vi "MegaAwesome_9_21_12c_JW.vi"() -> ()   [LabVIEW 2011]
uses:
  MegaAwesome_States.ctl
  <vilib>/Utility/inputDevices.llb/keyboardAcquire.vi
  <vilib>/Utility/file.llb/Read From Spreadsheet File (string).vi
  <vilib>/Utility/file.llb/Write To Spreadsheet File (string).vi
panel:
  out "Image Center X":i32
  in  "Disable Flag":bool
  out "Index":string
  out "ROI Descriptor out":T1 {"Contours"."Type" items=["No Selection", "Point", "Line", "Rectangle", "Oval", "Polygon", "Freehand Region", "Annulus", "Unused2", "Unused3", "Broken Line", "Freehand Line", "Rotated Rectangle"]}
  out "ROI Descriptor":T1 {"Contours"."Type" items=["No Selection", "Point", "Line", "Rectangle", "Oval", "Polygon", "Freehand Region", "Annulus", "Unused2", "Unused3", "Broken Line", "Freehand Line", "Rotated Rectangle"]}
  in  "Slider Min":dbl=5.0
  in  "Slider Max":dbl=5.0
  out "Opj X Axis":string
  out "X Axis Display Type":string
  in  "Index-Sat":dbl=5.0
  in  "Index-Lin":dbl=5.0
  in  "IndexLog-Lin":dbl=5.0
  in  "IndexLog-Sat":dbl=5.0 caption="Num Pts"
  out "Lin Id-Log Used":dbl[](array[numeric])
  out "Lin-Vg Array-Log Used":dbl[](array[numeric])
  in  "New: Comments":string
  out "Save Array":string[][](array[string])
  out "Folder Index":i32 caption="Length"
  out "Sat Id-Used":dbl[](array[numeric])
  out "Sat Vg Array-Used":dbl[](array[numeric])
  out "Vg Array-Log-Used":dbl[](array[numeric])
  out "Sat Id-Log-Used":dbl[](array[numeric])
  out "Lin Id-Used":dbl[](array[numeric])
  out "Lin-Vg Array-Used":dbl[](array[numeric])
  out "Lin Vd":dbl
  out "Recorded Prop":T2
  out "Current State":T3
  in  "Main Tab Control":T4(tab)
  in  "1) Transport":bool caption="2) Transport"
  in  "Image Analysis":bool caption="1) Image Analysis"
  in  "Transport\nFolder":path caption="Transport Folder"
  out "Transport\nFile":path=path "D:/UserData/Desktop/Jeremy/WFU/Research/Programs/VI mods/Image Not Found.png" caption="Transport File"
  in  "Image Folder":path
  out "Image File":path=path "D:/UserData/Desktop/Jeremy/WFU/Research/Programs/VI mods/Image Not Found.png"
  in  "Transfer File":path
  out "Transfer Folder":path
  out "Fabrication Prop":T5
  out "Distances":dbl[](array[numeric])
  in  "Zoom":i16(slide)=-3 scale=-5.0..5.0
  in  "Magnification":u16(ring) items=["5x", "10x", "20x", "50x", "80x"]
  in  "Undo Button":bool
  in  "Remove Button":bool
  in  "Transfer Plots":T6(tab)=enum."Saturation"
  in  "Lin-Trans Slider":dbl(slide) step=1.0 scale=-40.0..40.0 scale format="%#_1p"
  out "Sqrt-Lin":cluster{dbl[], dbl[]}[](graph)
  in  "Sat-Trans Slider":dbl(slide) step=1.0 scale=-40.0..40.0 scale format="%#_1p"
  out "Sqrt-Sat":cluster{dbl[], dbl[]}[](graph)
  out "Raw- Lin":cluster{dbl[], dbl[]}[](graph)
  out "Raw- Sat":cluster{dbl[], dbl[]}[](graph)
  in  "Log Plots":enum32{"Linear", "Saturation", "Transport"}(tab)=enum."Saturation"
  in  "Lin-Log Slider":dbl(slide) step=1.0 scale=-40.0..40.0 scale format="%#_1p"
  out "Log-Lin":cluster{dbl[], dbl[]}[](graph)
  in  "Sat-Log Slider":dbl(slide) step=1.0 scale=-40.0..40.0 scale format="%#_1p"
  out "Sat-Log":cluster{dbl[], dbl[]}[](graph)
  out "Transport":cluster{dbl[], dbl[]}[](graph)
  out "Transport Name:":string
  in  "Manual Controls":T7
  in  "File Controls":T8
  out "Date Recorded":string="Date Recorded" caption="Measured"
  out "Data Name:":string
  out "Image Name":string
  out "Date Created":string caption="Fabricated"
  in  "Comments:":string
  out "Rec: Length":dbl caption="Length" format="%#_3g"
  out "Rec: Width":dbl caption="Width" format="%#_4g"
  out "Rec: Dielectric (d)":dbl caption="Dielectric (d)" format="%#_3g"
  in  "New: Dielectric":dbl
  in  "New: Length":dbl
  in  "New: Width":dbl
  out "Rec: Temp":dbl caption="Sample Temp" format="%.1f"
  in  "New: Temp":dbl format="%.1f"
  out "Image Out":T9(plugin-control)
  in  "Num Pts":dbl=5.0
  in  "Num Pts Log":dbl=5.0 caption="Num Pts"
  out "Recorded Values Cluster":T10
  out "Calculated Values Cluster":T10 caption="Recorded Values Cluster"
  out "Re-Calculated Values Cluster":T10 caption="Recorded Values Cluster"
  in  "Independant Variable:":string(combo)="Length (um):"
  out "Image Preview":T9(plugin-control)
  out "Total Width":dbl
  in  "Index Array":u16(ring) caption="Index" items=["X 1B", "X 1C", "X 1D", "X 1E", "X 1F", "X 1H", "X 1J", "X 2A", "X 2B", "X 2C", "X 2D", "X 2E", "X 2F", "X 2G", "X 2H", "X 2J", "X 3A", "X 3B", "X 3C", "X 3D", "X 3E", "X 3F", "X 3G", "X 3H", "X 3J", "X 4A", "X 4B", "X 4C", "X 4D", "X 4E", "X 4F", "X 4G", "X 4H", "X 4J", "X 5A", "X 5B", "X 5C", "X 5D", "X 5E", "X 5F", "X 5G", "X 5H", "X 5J", "X 6A", "X 6B", "X 6C", "X 6D", "X 6E", "X 6F", "X 6G", "X 6H", "X 6J", "X 7A", "X 7B", "X 7C", "X 7D", "X 7E", "X 7F", "X 7G", "X 7J", "X 8A", "X 8B", "X 8C", "X 8D", "X 8E", "X 8F", "X 8G", "X 8H", "X 8J", "X 9C", "X 9D", "X F_"]
  in  "Room Temp":dbl=294.0 caption="Room Temp (K)"
  in  "No Image\n File":path=path "\\\\acad1\\physics/Jurchescu-group/JW-PD/Mega Awesome/Image Not Found.png" caption="No Image File"
  in  "Origin Project File":path=path "\\\\acad1\\physics/Jurchescu-group/JW-PD/Group Library/Origin Project Files/DeviceData_8_10_12a_JW.opj"
  in  "No Transport\n File":path=path "\\\\acad1\\physics/Jurchescu-group/JW-PD/Mega Awesome/No Transport File.txt" caption="No Transport File"
  in  "Transport Style Controls":T11={"Transport Line Size"=1, "Transport Line Color"=16772608} {"Transport Line Size" items=["Extra Small", "Small", "Medium", "Large", "Extra Large"]}
  # "Transfer Location"
  # "What else would you like to view during your analysis?"
  # "Image Location"
  # "Transport Location"
  # "Recorded"
  # "Calculated"
  # "Re-Calculated"
  # "Manual"
  # "Used points display at y=0\nValues are wrong w/ slider"
  # "Slider\nDoesn't\nWork"
  # "Slider\nDoesn't\nWork"
  # "No new points displayed"
  # "Default File Choices"
  # "Default Analysis Values"
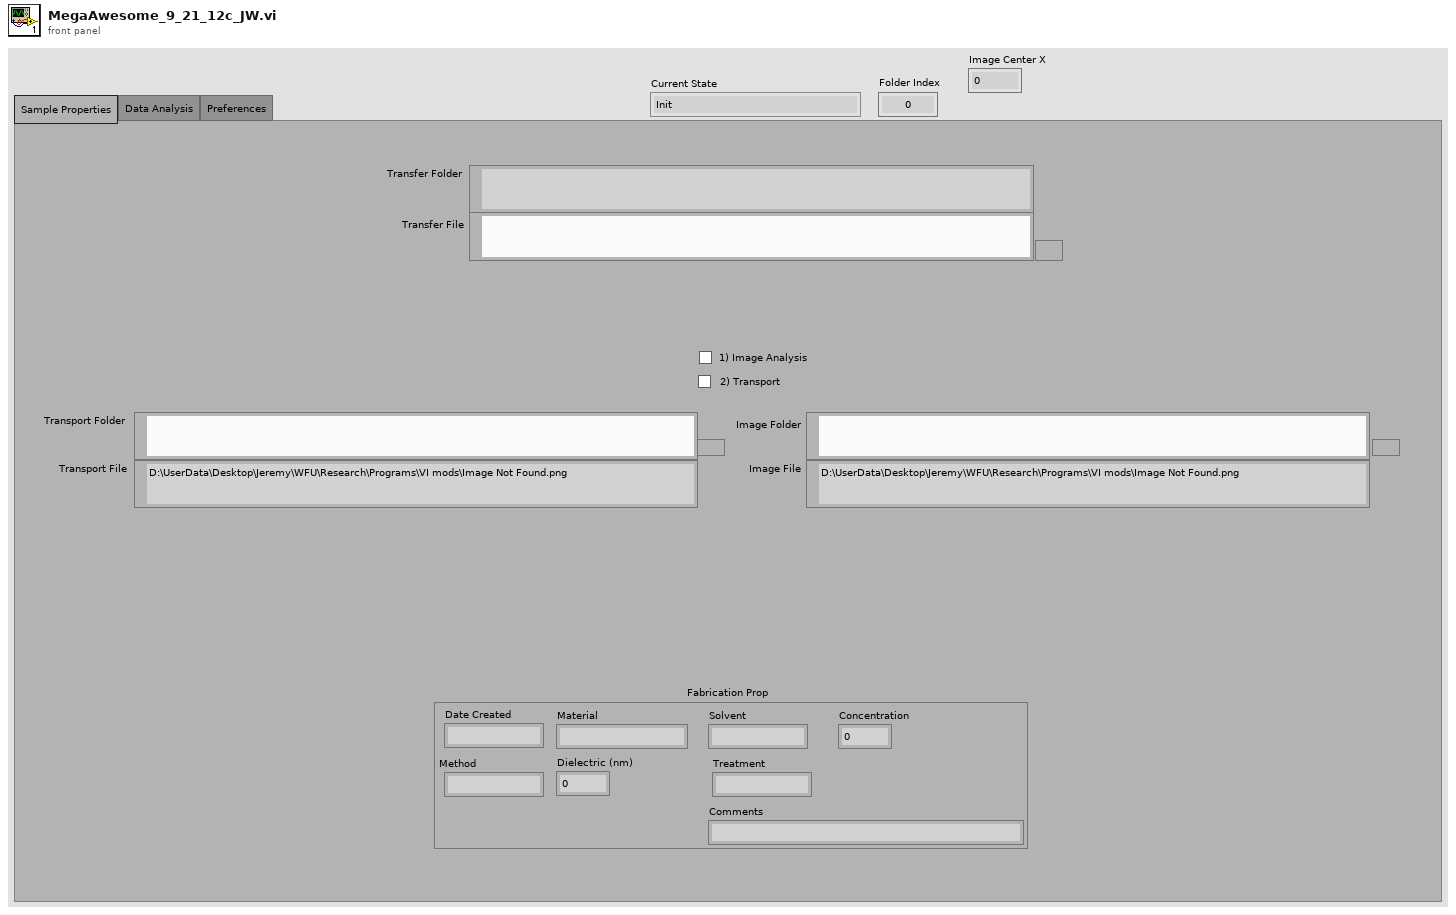
[diagram p1: front panel]
types:
  T1 = typedef "ROI Descriptor" = cluster{"Global Rectangle":i32[], "Contours":cluster{"ID":enum32{"External", "Internal"}, "Type":u32, "Coordinates":i32[]}[]}
  T2 = cluster{"Date Recorded":string, "Index":string, "Length":dbl, "Width":dbl, "Sample Temp":dbl}
  T3 = typedef "MegaAwesome_States.ctl" = enum16{"Init", "File Missing", "No Event", "Read Data", "Calculated Values", "Re-Calculated Values", "Next File", "Previous File", "Discard File", "Save", "Save Lines", "Export", "Exit"}
  T4 = enum32{"Sample Properties", "Data Analysis", "Preferences"}
  T5 = cluster{"Date Created":string, "Material":string, "Solvent":string, "Concentration":dbl, "Method":string, "Dielectric (nm)":dbl, "Treatment":string, "Comments":string}
  T6 = enum32{"Linear", "Saturation", "Raw-Linear", "Raw-Saturation"}
  T7 = cluster{"Manual-Temp":bool, "Manual-Width":bool, "Manuel-Length":bool, "Manuel-Dielectric":bool, "Manual Comments":bool}
  T8 = cluster{"Previous File":bool, "Discard ":bool, "Save Lines":bool, "Close":bool, "Next File ":bool, "Save":bool, "Save Next":bool, "Export":bool}
  T9 = typedef "IMAQ Image.ctl" = refnum<image>
  T10 = cluster{"Mobility-Sat":dbl, "Moblitity-Lin":dbl, "On/Off":dbl, "Off Current":dbl, "Vt-Sat":dbl, "STS":dbl, "Trap Density-VT":dbl, "Trap Density-STS":dbl}
  T11 = cluster{"Transport Line Size":u16, "Transport Line Color":u32}
  T12 = typedef "LVBoundsTypeDef.ctl" = cluster{"Width":u32, "Height":u32}
  T13 = cluster{"Global Rectangle":i32[], "Contours":cluster{"Contour Type":u32, "ROI Type":u32, "Points":i32[]}[]}
  T14 = cluster{"Contour Type":u32, "ROI Type":u32, "Points":i32[]}[]
  T15 = cluster{i32[], cluster{"Contour Type":u32, "ROI Type":u32, "Points":i32[]}[]}
  T16 = enum16{"0", "1", "2", "3", "4", "5", "6", "7", "8", "9", "A", "B", "C", "D", "E", "F", "G", "H", "I", "J", "K", "L", "M", "N", "O", "P", "Q", "R", "S", "T", "U", "V", "W", "X", "Y", "Z", "F1", "F2", "F3", "F4", "F5", "F6", "F7", "F8", "F9", "F10", "F11", "F12", "F13", "F14", "F15", "ADD", "BACK", "BACKSLASH", "CAPITAL", "COMMA", "DECIMAL", "DELETE", "DIVIDE", "DOWN", "END", "EQUALS", "ESCAPE", "GRAVE (`)", "HOME", "INSERT", "LBRACKET", "LCONTROL", "LEFT", "L ALT", "LSHIFT", "LWIN", "MINUS", "MULTIPLY", "NEXT", "NUMLOCK", "NUMPAD_0", "NUMPAD_1", "NUMPAD_2", "NUMPAD_3", "NUMPAD_4", "NUMPAD_5", "NUMPAD_6", "NUMPAD_7", "NUMPAD_8", "NUMPAD_9", "PAUSE", "PERIOD", "PRIOR (PG UP)", "RBRACKET", "RCONTROL", "RETURN", "RIGHT", "R ALT", "RSHIFT", "RWIN", "SCROLL", "SEMICOLON", "SLASH", "SPACE", "SUBTRACT", "TAB", "UP", "ENTER (num pad)", "' (quote)"}[]
  T17 = enum16{"0", "1", "2", "3", "4", "5", "6", "7", "8", "9", "A", "B", "C", "D", "E", "F", "G", "H", "I", "J", "K", "L", "M", "N", "O", "P", "Q", "R", "S", "T", "U", "V", "W", "X", "Y", "Z", "F1", "F2", "F3", "F4", "F5", "F6", "F7", "F8", "F9", "F10", "F11", "F12", "F13", "F14", "F15", "ADD", "BACK", "BACKSLASH", "CAPITAL", "COMMA", "DECIMAL", "DELETE", "DIVIDE", "DOWN", "END", "EQUALS", "ESCAPE", "GRAVE (`)", "HOME", "INSERT", "LBRACKET", "LCONTROL", "LEFT", "L ALT", "LSHIFT", "LWIN", "MINUS", "MULTIPLY", "NEXT", "NUMLOCK", "NUMPAD_0", "NUMPAD_1", "NUMPAD_2", "NUMPAD_3", "NUMPAD_4", "NUMPAD_5", "NUMPAD_6", "NUMPAD_7", "NUMPAD_8", "NUMPAD_9", "PAUSE", "PERIOD", "PRIOR (PG UP)", "RBRACKET", "RCONTROL", "RETURN", "RIGHT", "R ALT", "RSHIFT", "RWIN", "SCROLL", "SEMICOLON", "SLASH", "SPACE", "SUBTRACT", "TAB", "UP", "ENTER (num pad)", "' (quote)"}
  T18 = cluster{string, sgl, bool, bool, bool, bool, bool, bool, i32}
  T19 = cluster{i32, cluster{string, sgl, bool, bool, bool, bool, bool, bool, i32}, i32, i32}
  T20 = cluster{"Contour Type":u32, "ROI Type":u32, "Points":i32[]}
  T21 = cluster{"Points[0]":i32, "Points[1]":i32, "Points[2]":i32, "Points[3]":i32, "Points[4]":i32, "Points[5]":i32, "Points[6]":i32, "Points[7]":i32, "Points[8]":i32}
  T22 = cluster{"[0]":cluster{dbl[], dbl[]}, "[1]":cluster{dbl[], dbl[]}, "[2]":cluster{dbl[], dbl[]}, "[3]":cluster{dbl[], dbl[]}, "[4]":cluster{dbl[], dbl[]}, "[5]":cluster{dbl[], dbl[]}, "[6]":cluster{dbl[], dbl[]}, "[7]":cluster{dbl[], dbl[]}, "[8]":cluster{dbl[], dbl[]}}
  T23 = cluster{"Sat Vg Used":dbl[], "Sat Sqrt(Id) Used ":dbl[], "Lin Vg Used":dbl[], "Lin Sqrt(Id) Used":dbl[], "Index-Lin":dbl, "Index-Sat":dbl}
  T24 = cluster{"Raw Sat":cluster{dbl[], dbl[]}[], "Sqrt Sat":cluster{dbl[], dbl[]}[], "Log Sat":cluster{dbl[], dbl[]}[], "Raw Lin":cluster{dbl[], dbl[]}[], "Sqrt Lin":cluster{dbl[], dbl[]}[], "Log Lin":cluster{dbl[], dbl[]}[]}
  T25 = cluster{"Mobility-Sat":dbl, "Vt-Sat":dbl, "Mobility-Lin":dbl, "Vt-Lin":dbl, "Off I-Sat":dbl, "On/Off I-Sat":dbl}
  T26 = cluster{"Sat Vg Used":dbl[], "Sat Log(Id) Used":dbl[], "Lin Vg Used":dbl[], "Lin Log(Id) Used":dbl[], "STS Index-Sat":dbl, "STS Index-Lin":dbl}
  T27 = cluster{"Independant  Variable Indicator":string, "Parameter String Indicator":string}
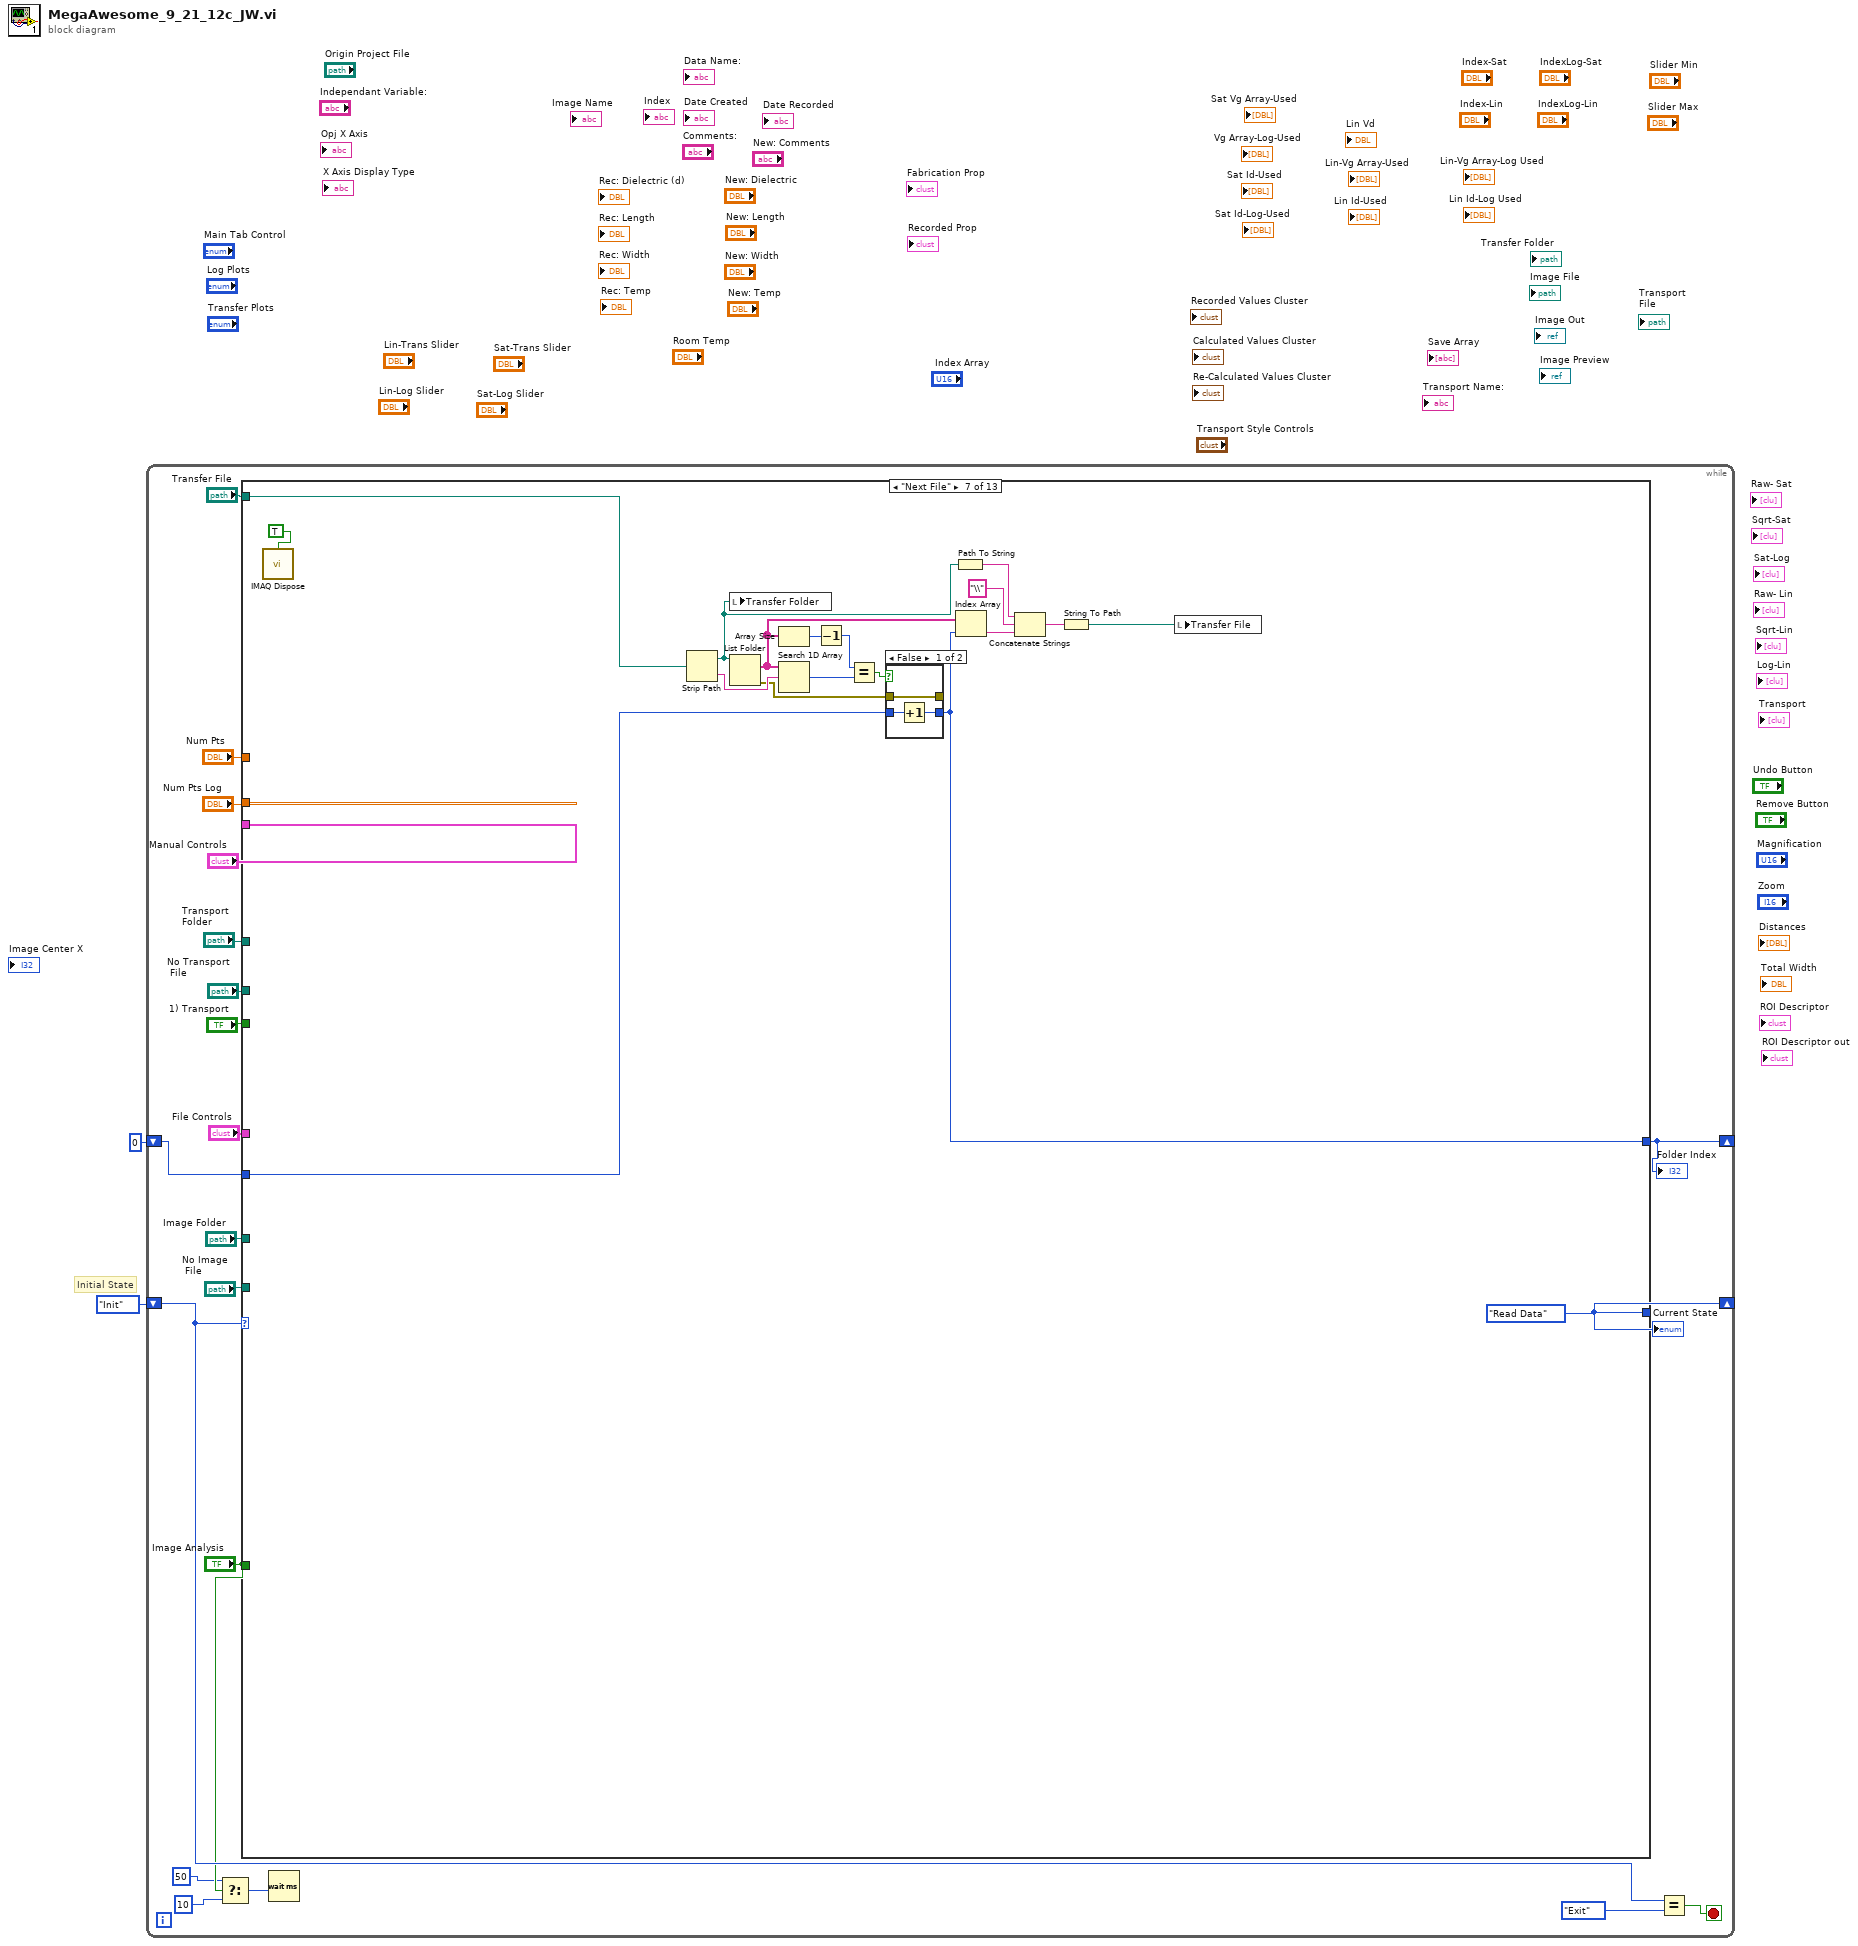
[diagram p0: block diagram]
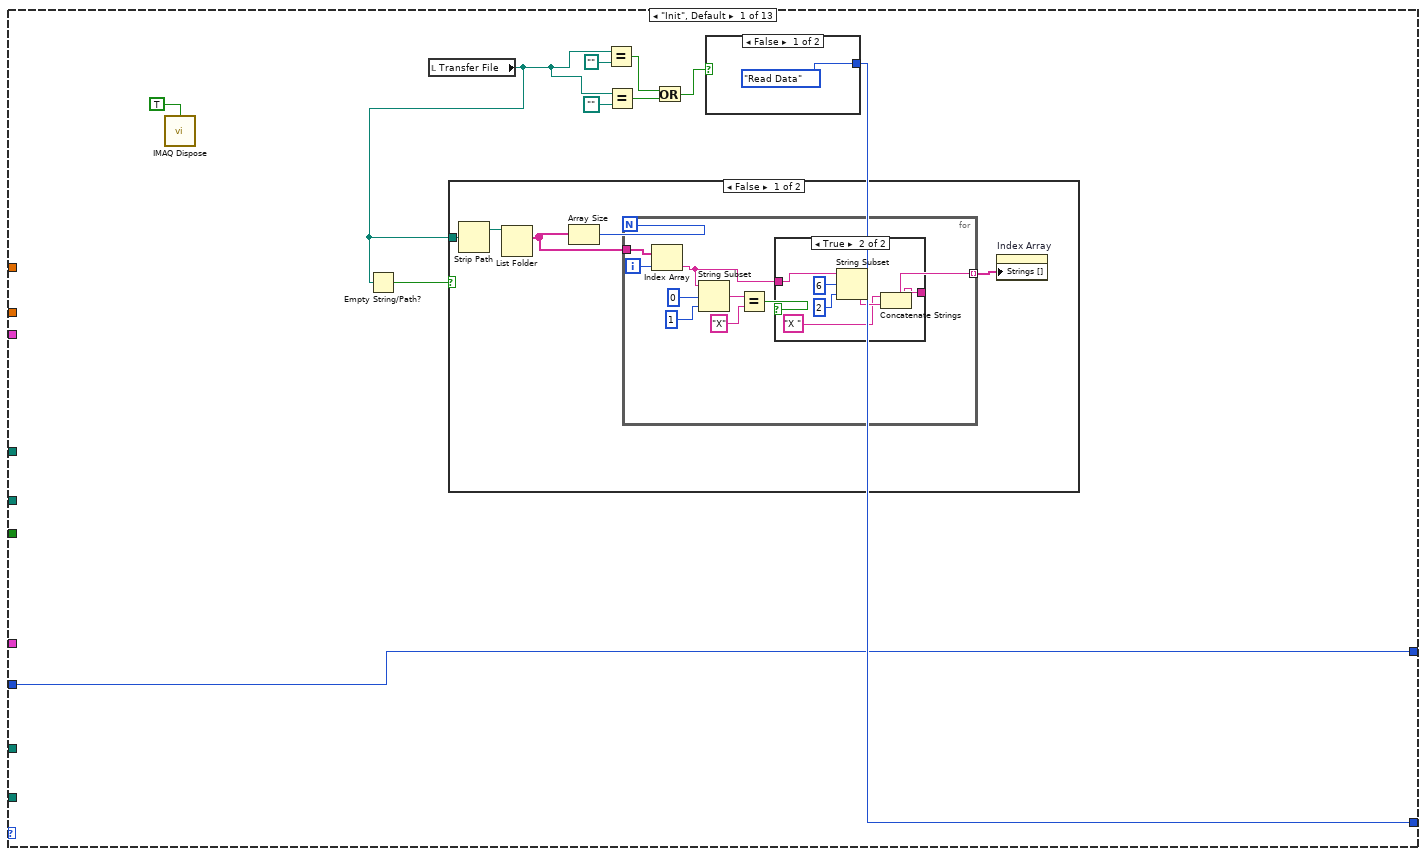
[diagram p2: hidden frame]
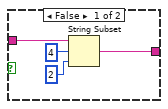
[diagram p3: hidden frame]
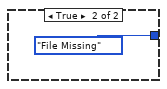
[diagram p5: hidden frame]
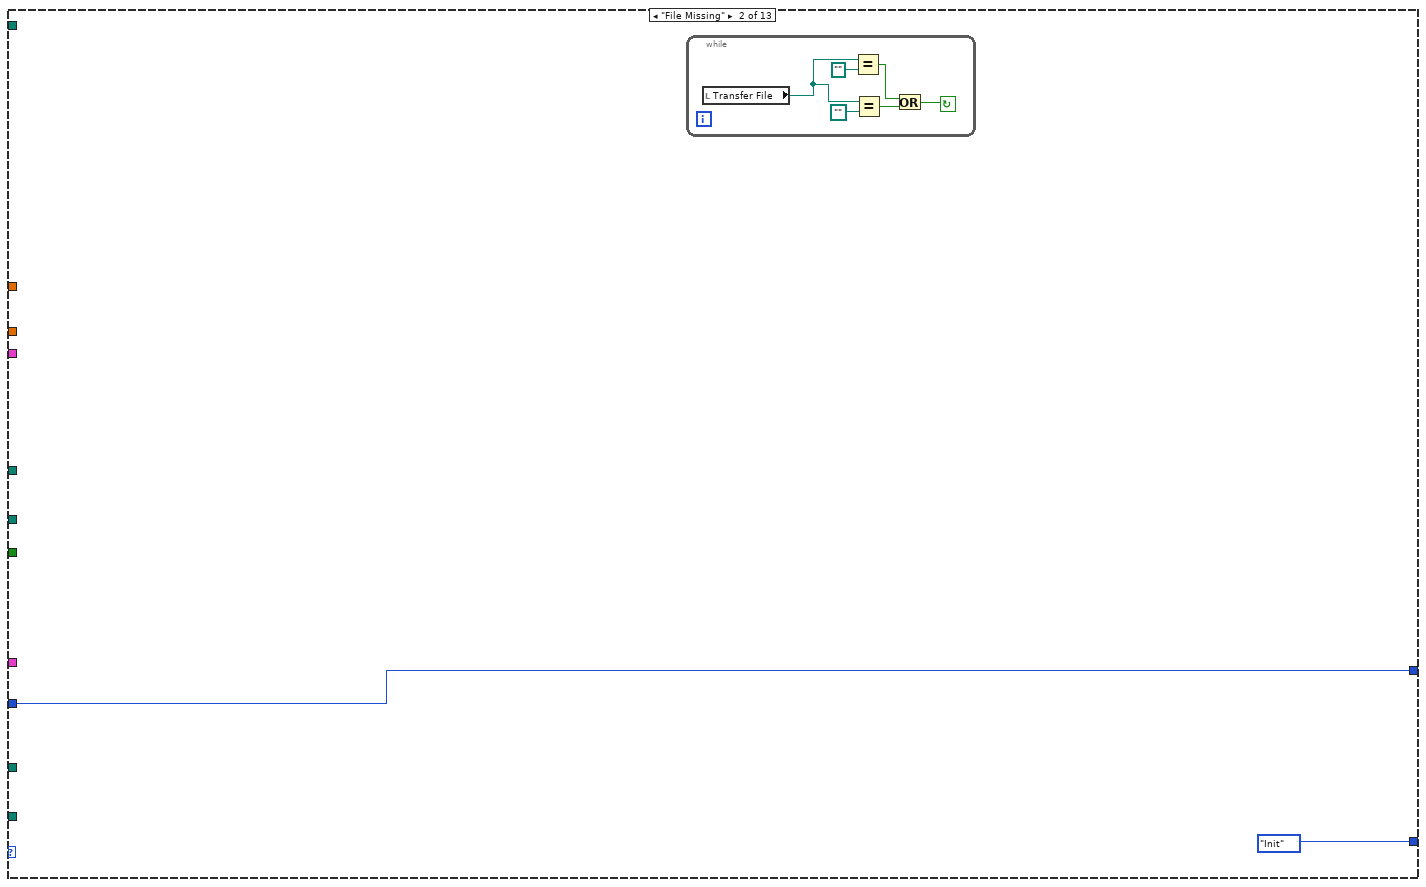
[diagram p6: hidden frame]
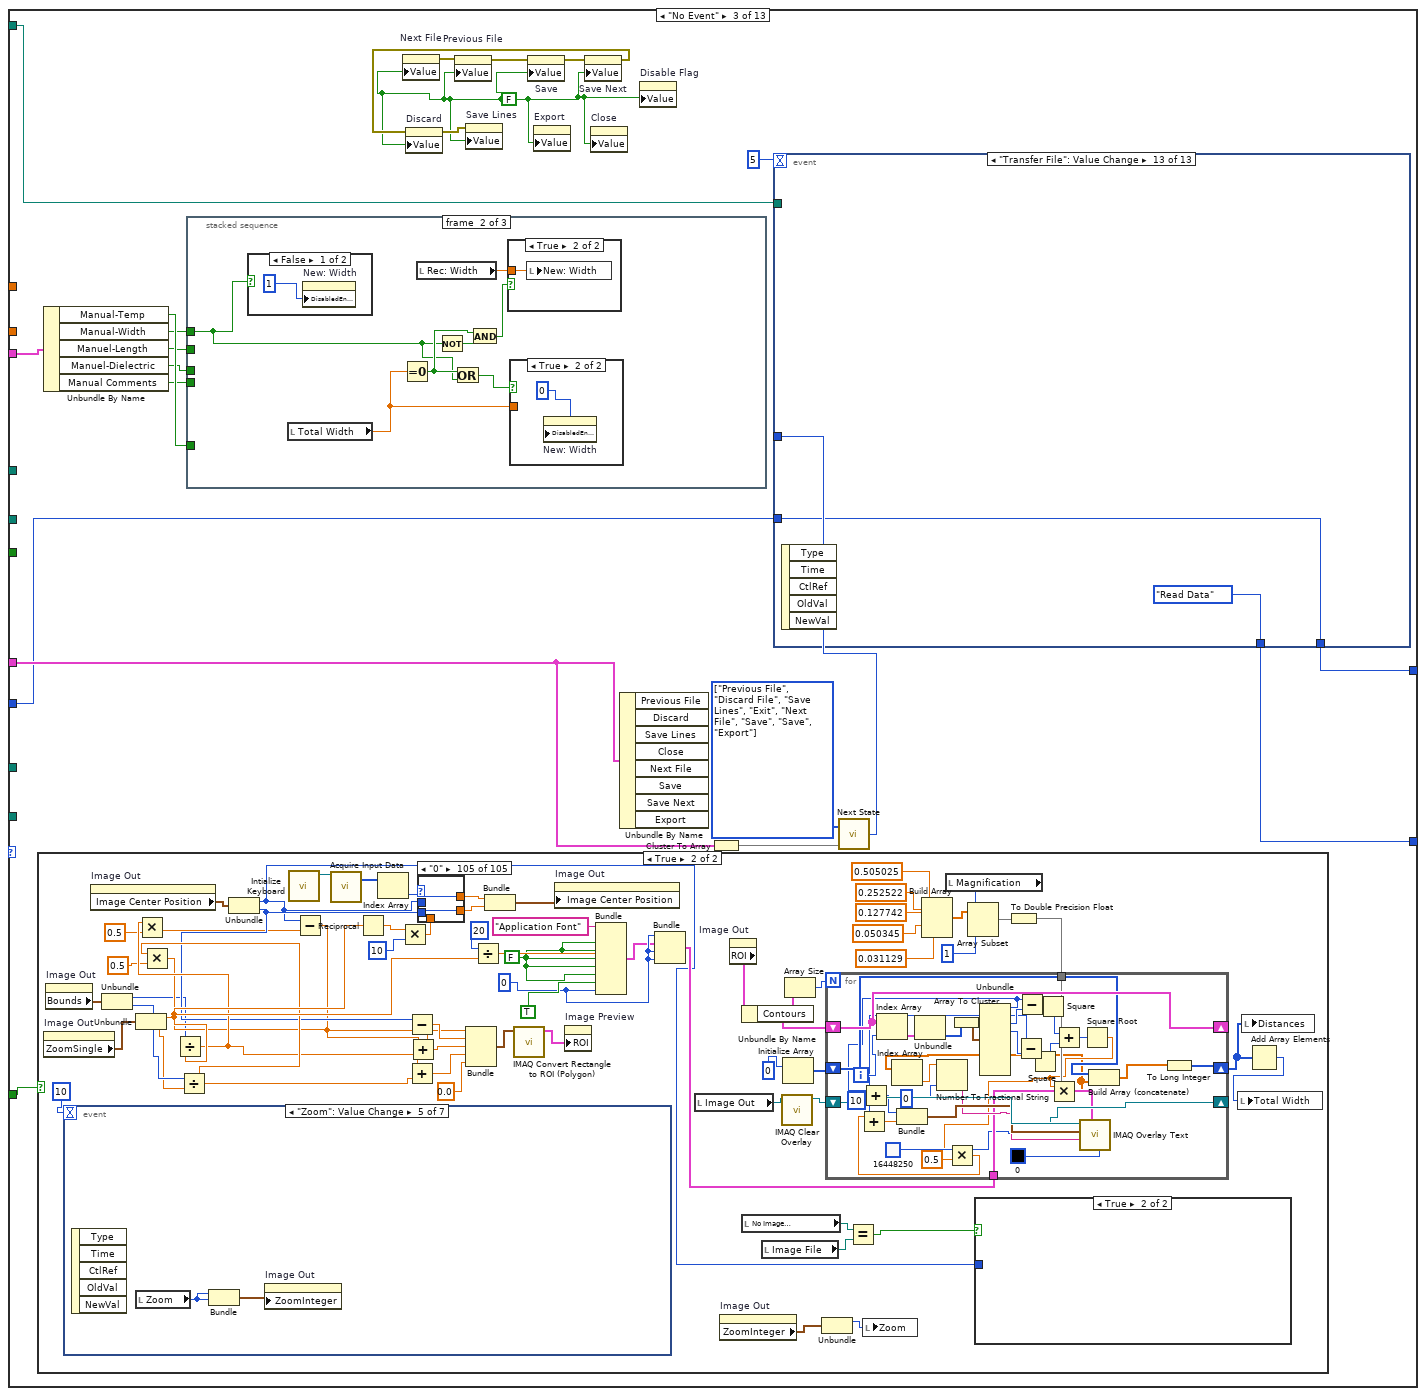
[diagram p7: hidden frame]
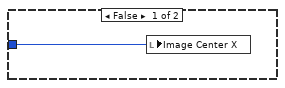
[diagram p9: hidden frame]
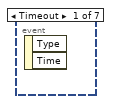
[diagram p10: hidden frame]
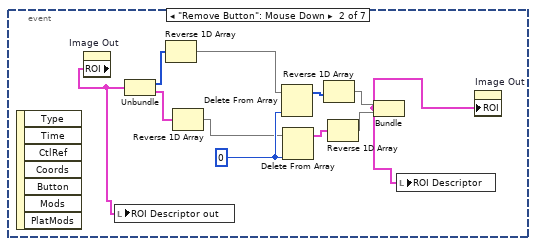
[diagram p11: hidden frame]
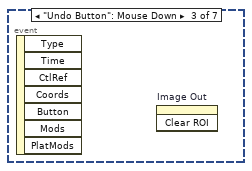
[diagram p12: hidden frame]
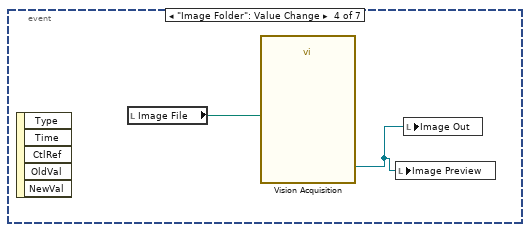
[diagram p13: hidden frame]
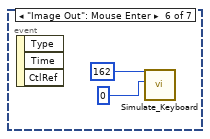
[diagram p14: hidden frame]
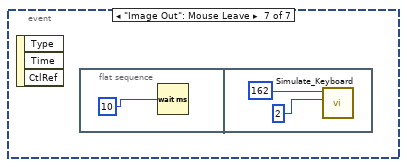
[diagram p15: hidden frame]
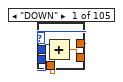
[diagram p16: hidden frame]
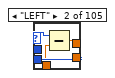
[diagram p17: hidden frame]
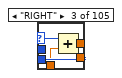
[diagram p18: hidden frame]
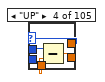
[diagram p19: hidden frame]
diagram:
  # "Initial State"
  n1 = while {
    shift-right: [w19] -> _
    shift-left: MegaAwesome_States."Init" -> [w21]
    shift-right: [w12] -> _
    shift-left: 0 -> [w13]
    stop <- w22 stop-if-true
    n2 = Select(t=50, s="Image Analysis", f=10) -> (s? t:f=w6:i32)
    n3 = case shown="\"Next File\"" w21 {
      tunnel: [w27 MegaAwesome_States."Init" w79 MegaAwesome_States."Calculated Values" MegaAwesome_States."Re-Calculated Values" MegaAwesome_States."No Event" MegaAwesome_States."Read Data" MegaAwesome_States."Read Data" MegaAwesome_States."Init" w813 MegaAwesome_States."No Event" MegaAwesome_States."No Event" MegaAwesome_States."Exit"] -> w19
      tunnel: "Transfer File" -> [_ _ w68 w578 w628 _ w750 w763 w784 w818 _ _ _]
      tunnel: "Num Pts" -> [_ _ _ _ w652 _ _ _ _ _ _ _ _]
      tunnel: "Num Pts Log" -> [_ _ _ _ w651 _ _ _ _ _ _ _ _]
      tunnel: "Image Folder" -> [_ _ _ _ w648 _ _ _ _ _ _ w1337 _]
      tunnel: "No Image\n File" -> [_ _ _ _ w647 _ _ _ _ _ _ _ _]
      tunnel: [w26 w59 w69 w583 w646 w709 w735 w761 w779 w819 w1334 w1347 w1351] -> w12
      tunnel: w13 -> [w26 w59 w70 w581 w646 w709 w736 w762 _ w819 w1334 w1347 w1351]
      tunnel: "Manual Controls" -> [_ _ w81 _ _ _ _ _ _ w817 _ _ _]
      tunnel: "File Controls" -> [_ _ w77 _ _ _ _ _ _ w812 _ _ _]
      tunnel: "1) Transport" -> [_ _ _ _ w618 _ _ _ _ _ _ _ _]
      tunnel: "Image Analysis" -> [_ _ w71 _ w617 _ _ _ _ _ _ _ _]
      tunnel: "Transport\nFolder" -> [_ _ _ _ w616 _ _ _ _ _ _ _ _]
      tunnel: "No Transport\n File" -> [_ _ _ _ w615 _ _ _ _ _ _ _ _]
      frame "Init", Default {
        n4 = call "IMAQ Dispose"("All Images? (No)"=TRUE) -> ()  [unwired: 5 in, 1 out]
        n5 = local read "Transfer File"() -> (w24:path)
        n6 = Empty String/Path?(string/path=w24) -> (empty?=w25:bool)
        n7 = case shown="False" w25 {
          tunnel: w24 -> [w34 _]
          frame False {
            n8 = Strip Path(path=w34) -> (stripped path=w36:path)  [unwired: 1 out]
            n9 = List Folder(path=w36) -> (filenames=w35:string[])  [unwired: 3 in, 3 out]
            n10 = Array Size(array=w35) -> (size(s)=w37:i32)
            n11 = for {
              N: w37 -> [_]
              tunnel: w35 -> [w46]
              tunnel: [w44] -> w33 mode=indexing
              i -> [w45]
              n12 = Index Array(array=w46, index=w45) -> (element=w43:string)
              n13 = String Subset(string=w43, offset (0)=0, length (rest)=1) -> (substring=w40:string)
              n14 = Equal?(x=w40, y="X") -> (x = y?=w39:bool)
              n15 = case shown="True" w39 {
                tunnel: w43 -> [w50 w54]
                tunnel: [w47 w53] -> w44
                frame False {
                  n16 = String Subset(string=w50, offset (0)=4, length (rest)=2) -> (substring=w47:string)
                }
                frame True {
                  n17 = String Subset(string=w54, offset (0)=6, length (rest)=2) -> (substring=w52:string)
                  n18 = Concatenate Strings("X ", w52) -> (w53:string)
                }
              }
            }
            n19 = property on="Index Array" class="Ring (strict)"("Strings []"=w33) -> ()  [unwired: 2 in, 2 out]
          }
          frame True {
          }
        }
        n20 = Equal?(x=w24, y=path "") -> (x = y?=w30:bool)
        n21 = Equal?(x=w24, y=path "") -> (x = y?=w29:bool)
        n22 = Or(x=w30, y=w29) -> (x .or. y?=w32:bool)
        n23 = case shown="False" w32 {
          tunnel: [MegaAwesome_States."Read Data" MegaAwesome_States."File Missing"] -> w27
          frame False {
          }
          frame True {
          }
        }
      }
      frame "File Missing" {
        n24 = while {
          stop <- w61 continue-if-true
          n25 = local read "Transfer File"() -> (w62:path)
          n26 = Equal?(x=w62, y=path "") -> (x = y?=w64:bool)
          n27 = Equal?(x=w62, y=path "") -> (x = y?=w65:bool)
          n28 = Or(x=w64, y=w65) -> (x .or. y?=w61:bool)
        }
      }
      frame "No Event" {
        w67 = FALSE
        w88 = T3[] [enum."Previous File", enum."Discard File", enum."Save Lines", enum."Exit", enum."Next File", enum."Save", enum."Save", enum."Export"] items=["Init", "File Missing", "No Event", "Read Data", "Calculated Values", "Re-Calculated Values", "Next File", "Previous File", "Discard File", "Save", "Save Lines", "Export", "Exit"]
        n29 = case shown="True" w71 {
          frame False {
          }
          frame True {
            w144 = FALSE
            w146 = 0
            n30 = property on="Image Out" class="ImageControl"() -> ("ZoomSingle"=w130:cluster{"X":sgl, "Y":sgl})  [unwired: 2 in, 2 out]
            n31 = property on="Image Out" class="ImageControl"() -> ("Bounds"=w129:T12)  [unwired: 2 in, 2 out]
            n32 = event shown="[4] \"Zoom\": Value Change" {
              selector: _ -> [_ _ _ _ _ _ _]
              dyn-events: _ -> [_ _ _ _ _ _ _]
              timeout: 10 -> [_ _ _ _ _ _ _]
              event Timeout {
                n33 = event-data() -> ()  [unwired: 1 in, 2 out]
              }
              event "Remove Button": Mouse Down {
                w164 = 0
                n34 = event-data() -> ()  [unwired: 1 in, 7 out]
                n35 = property on="Image Out" class="ImageControl"() -> ("ROI"=w154:T13)  [unwired: 2 in, 2 out]
                n36 = local write "ROI Descriptor out"(w154) -> ()
                n37 = Unbundle(w154) -> ("Global Rectangle"=w163:i32[], "Contours"=w161:T14)
                n38 = Reverse 1D Array(array=w163) -> (reversed array=w162:i32[])
                n39 = Reverse 1D Array(array=w161) -> (reversed array=w160:T14)
                n40 = Delete From Array(array=w162, index=w164) -> (array with subset deleted=w159:i32[])  [unwired: 1 in, 1 out]
                n41 = Delete From Array(array=w160, index=w164) -> (array with subset deleted=w158:T14)  [unwired: 1 in, 1 out]
                n42 = Reverse 1D Array(array=w159) -> (reversed array=w157:i32[])
                n43 = Reverse 1D Array(array=w158) -> (reversed array=w156:T14)
                n44 = Bundle(w157, w156) -> (w155:T15)  [unwired: 1 in]
                n45 = local write "ROI Descriptor"(w155) -> ()
                n46 = property on="Image Out" class="ImageControl"("ROI"=w155) -> ()  [unwired: 2 in, 2 out]
              }
              event "Undo Button": Mouse Down {
                n47 = event-data() -> ()  [unwired: 1 in, 7 out]
                n48 = invoke on="Image Out" class="ImageControl" method="Clear ROI"() -> ()  [unwired: 3 in, 3 out]
              }
              event "Image Folder": Value Change {
                n49 = event-data() -> ()  [unwired: 1 in, 5 out]
                n50 = local read "Image File"() -> (w166:path)
                n51 = call "Vision Acquisition"("Image Path"=w166) -> ("Image Out"=w165:T9)  [unwired: 25 in, 1 out]
                n52 = local write "Image Preview"(w165) -> ()
                n53 = local write "Image Out"(w165) -> ()
              }
              event "Zoom": Value Change {
                n54 = event-data() -> ()  [unwired: 1 in, 5 out]
                n55 = local read "Zoom"() -> (w167:i16)
                n56 = Bundle("Zoom"=w167, "Zoom"=w167) -> (w168:cluster{"Zoom":i16, "Zoom":i16})  [unwired: 1 in]
                n57 = property on="Image Out" class="ImageControl"("ZoomInteger"=w168) -> ()  [unwired: 2 in, 2 out]
              }
              event "Image Out": Mouse Enter {
                n58 = event-data() -> ()  [unwired: 1 in, 3 out]
                n59 = call "Simulate_Keyboard.vi"("Action"=0, "Virtual Key"=162) -> ()  [unwired: 7 in, 1 out]
              }
              event "Image Out": Mouse Leave {
                n60 = event-data() -> ()  [unwired: 1 in, 3 out]
                n61 = flat-sequence {
                  frame #0 {
                    n62 = Wait (ms)(milliseconds to wait=10) -> ()  [unwired: 1 out]
                  }
                  frame #1 {
                    n63 = call "Simulate_Keyboard.vi"("Action"=2, "Virtual Key"=162) -> ()  [unwired: 7 in, 1 out]
                  }
                }
              }
            }
            n64 = property on="Image Out" class="ImageControl"() -> ("Image Center Position"=w123:cluster{"X":u32, "Y":u32})  [unwired: 2 in, 2 out]
            n65 = Unbundle(w129) -> ("Width"=w132:u32, "Height"=w133:u32)
            n66 = Unbundle(w130) -> ("X"=w150:sgl, "Y"=w131:sgl)
            n67 = Divide(x=w132, y=w150) -> (x/y=w141:sgl)
            n68 = Multiply(x=w141, y=0.5) -> (x*y=w136:dbl)
            n69 = Divide(x=w133, y=w131) -> (x/y=w142:sgl)
            n70 = Multiply(x=w142, y=0.5) -> (x*y=w137:dbl)
            n71 = Unbundle(w123) -> ("X"=w92:u32, "Y"=w140:u32)
            n72 = call <vilib>:"Intialize Keyboard.vi"() -> ("device ID"=w120:refnum<k1>)  [unwired: 10 in, 1 out]
            n73 = Subtract(x=w92, y=w136) -> (x-y=w138:dbl)
            n74 = call-poly <vilib>:"Acquire Input Data.vi"("device ID"=w120) -> ("keys pressed"=w121:T16)  [unwired: 16 in, 2 out]
            n75 = Reciprocal(x=w150) -> (1/x=w151:sgl)
            n76 = Index Array(array=w121) -> (element=w117:T17)  [unwired: 1 in]
            n77 = Multiply(x=w151, y=10) -> (x*y=w149:sgl)
            n78 = Subtract(x=w140, y=w137) -> (x-y=w139:dbl)
            n79 = Add(x=w139, y=w142) -> (x+y=w125:dbl)
            n80 = Add(x=w138, y=w141) -> (x+y=w124:dbl)
            n81 = case shown="\"0\"" w117 {
              tunnel: w92 -> [w209 w215 w219 w221 w225 w227 w229 w231 w233 w235 w237 w239 w241 w243 w245 w247 w249 w251 w253 w255 w257 w259 w261 w263 w265 w267 w269 w271 w273 w275 w277 w279 w281 w283 w285 w287 w289 w291 w293 w295 w297 w299 w301 w303 w305 w307 w309 w311 w313 w315 w317 w319 w321 w323 w325 w327 w329 w331 w333 w335 w337 w339 w341 w343 w345 w347 w349 w351 w353 w355 w357 w359 w361 w363 w365 w367 w369 w371 w373 w375 w377 w379 w381 w383 w385 w387 w389 w391 w393 w395 w397 w399 w401 w403 w405 w407 w409 w411 w413 w415 w417 w419 w421 w423 w425]
              tunnel: [w209 w214 w218 w221 w225 w227 w229 w231 w233 w235 w237 w239 w241 w243 w245 w247 w249 w251 w253 w255 w257 w259 w261 w263 w265 w267 w269 w271 w273 w275 w277 w279 w281 w283 w285 w287 w289 w291 w293 w295 w297 w299 w301 w303 w305 w307 w309 w311 w313 w315 w317 w319 w321 w323 w325 w327 w329 w331 w333 w335 w337 w339 w341 w343 w345 w347 w349 w351 w353 w355 w357 w359 w361 w363 w365 w367 w369 w371 w373 w375 w377 w379 w381 w383 w385 w387 w389 w391 w393 w395 w397 w399 w401 w403 w405 w407 w409 w411 w413 w415 w417 w419 w421 w423 w425] -> w118
              tunnel: w140 -> [w211 w213 w217 w223 w224 w226 w228 w230 w232 w234 w236 w238 w240 w242 w244 w246 w248 w250 w252 w254 w256 w258 w260 w262 w264 w266 w268 w270 w272 w274 w276 w278 w280 w282 w284 w286 w288 w290 w292 w294 w296 w298 w300 w302 w304 w306 w308 w310 w312 w314 w316 w318 w320 w322 w324 w326 w328 w330 w332 w334 w336 w338 w340 w342 w344 w346 w348 w350 w352 w354 w356 w358 w360 w362 w364 w366 w368 w370 w372 w374 w376 w378 w380 w382 w384 w386 w388 w390 w392 w394 w396 w398 w400 w402 w404 w406 w408 w410 w412 w414 w416 w418 w420 w422 w424]
              tunnel: [w210 w213 w217 w222 w224 w226 w228 w230 w232 w234 w236 w238 w240 w242 w244 w246 w248 w250 w252 w254 w256 w258 w260 w262 w264 w266 w268 w270 w272 w274 w276 w278 w280 w282 w284 w286 w288 w290 w292 w294 w296 w298 w300 w302 w304 w306 w308 w310 w312 w314 w316 w318 w320 w322 w324 w326 w328 w330 w332 w334 w336 w338 w340 w342 w344 w346 w348 w350 w352 w354 w356 w358 w360 w362 w364 w366 w368 w370 w372 w374 w376 w378 w380 w382 w384 w386 w388 w390 w392 w394 w396 w398 w400 w402 w404 w406 w408 w410 w412 w414 w416 w418 w420 w422 w424] -> w119
              tunnel: w149 -> [w208 w212 w216 w220 _ _ _ _ _ _ _ _ _ _ _ _ _ _ _ _ _ _ _ _ _ _ _ _ _ _ _ _ _ _ _ _ _ _ _ _ _ _ _ _ _ _ _ _ _ _ _ _ _ _ _ _ _ _ _ _ _ _ _ _ _ _ _ _ _ _ _ _ _ _ _ _ _ _ _ _ _ _ _ _ _ _ _ _ _ _ _ _ _ _ _ _ _ _ _ _ _ _ _ _ _]
              frame "DOWN" {
                n82 = Add(x=w211, y=w208) -> (x+y=w210:sgl)
              }
              frame "LEFT" {
                n83 = Subtract(x=w215, y=w212) -> (x-y=w214:sgl)
              }
              frame "RIGHT" {
                n84 = Add(x=w219, y=w216) -> (x+y=w218:sgl)
              }
              frame "UP" {
                n85 = Subtract(x=w223, y=w220) -> (x-y=w222:sgl)
              }
              frame "ENTER (num pad)" {
              }
              frame "' (quote)" {
              }
              frame "END" {
              }
              frame "EQUALS" {
              }
              frame "ESCAPE" {
              }
              frame "GRAVE (`)" {
              }
              frame "HOME" {
              }
              frame "INSERT" {
              }
              frame "LBRACKET" {
              }
              frame "LCONTROL" {
              }
              frame "L ALT" {
              }
              frame "LSHIFT" {
              }
              frame "LWIN" {
              }
              frame "MINUS" {
              }
              frame "MULTIPLY" {
              }
              frame "NEXT" {
              }
              frame "NUMLOCK" {
              }
              frame "NUMPAD_0" {
              }
              frame "NUMPAD_1" {
              }
              frame "NUMPAD_2" {
              }
              frame "NUMPAD_3" {
              }
              frame "NUMPAD_4" {
              }
              frame "NUMPAD_5" {
              }
              frame "NUMPAD_6" {
              }
              frame "NUMPAD_7" {
              }
              frame "NUMPAD_8" {
              }
              frame "NUMPAD_9" {
              }
              frame "PAUSE" {
              }
              frame "PERIOD" {
              }
              frame "PRIOR (PG UP)" {
              }
              frame "RBRACKET" {
              }
              frame "RCONTROL" {
              }
              frame "RETURN" {
              }
              frame "R ALT" {
              }
              frame "RSHIFT" {
              }
              frame "RWIN" {
              }
              frame "SCROLL" {
              }
              frame "SEMICOLON" {
              }
              frame "SLASH" {
              }
              frame "SPACE" {
              }
              frame "SUBTRACT" {
              }
              frame "TAB" {
              }
              frame "DIVIDE" {
              }
              frame "DELETE" {
              }
              frame "DECIMAL" {
              }
              frame "COMMA" {
              }
              frame "CAPITAL" {
              }
              frame "BACKSLASH" {
              }
              frame "BACK" {
              }
              frame "ADD" {
              }
              frame "F15" {
              }
              frame "F14" {
              }
              frame "F13" {
              }
              frame "F12" {
              }
              frame "F11" {
              }
              frame "F10" {
              }
              frame "F9" {
              }
              frame "F8" {
              }
              frame "F7" {
              }
              frame "F6" {
              }
              frame "F5" {
              }
              frame "F4" {
              }
              frame "F3" {
              }
              frame "F2" {
              }
              frame "F1" {
              }
              frame "Z" {
              }
              frame "Y" {
              }
              frame "X" {
              }
              frame "W" {
              }
              frame "V" {
              }
              frame "U" {
              }
              frame "T" {
              }
              frame "S" {
              }
              frame "R" {
              }
              frame "Q" {
              }
              frame "P" {
              }
              frame "O" {
              }
              frame "N" {
              }
              frame "M" {
              }
              frame "L" {
              }
              frame "K" {
              }
              frame "J" {
              }
              frame "I" {
              }
              frame "H" {
              }
              frame "G" {
              }
              frame "F" {
              }
              frame "E" {
              }
              frame "D" {
              }
              frame "C" {
              }
              frame "B" {
              }
              frame "A" {
              }
              frame "9" {
              }
              frame "8" {
              }
              frame "7" {
              }
              frame "6" {
              }
              frame "5" {
              }
              frame "4" {
              }
              frame "3" {
              }
              frame "2" {
              }
              frame "1" {
              }
              frame "0" {
              }
            }
            n86 = Bundle(w138, w139, w124, w125, 0.0) -> (w126:cluster{dbl, dbl, dbl, dbl, dbl})  [unwired: 1 in]
            n87 = Divide(x=20, y=w150) -> (x/y=w148:sgl)
            n88 = Bundle("X"=w118, "Y"=w119) -> (w122:cluster{"X":sgl, "Y":sgl})  [unwired: 1 in]
            n89 = call "IMAQ Convert Rectangle to ROI (Polygon)"("Rectangle"=w126) -> ("ROI Descriptor"=w128:T1)  [unwired: 7 in, 2 out]
            n90 = property on="Image Out" class="ImageControl"("Image Center Position"=w122) -> ()  [unwired: 2 in, 2 out]
            n91 = property on="Image Preview" class="ImageControl"("ROI"=w128) -> ()  [unwired: 2 in, 2 out]
            n92 = Bundle("Application Font", w148, w144, w144, w144, w144, w144, TRUE, w146) -> (w143:T18)  [unwired: 1 in]
            n93 = Bundle(w146, w143, w146, w146) -> (w98:T19)  [unwired: 1 in]
            n94 = local read "Image Out"() -> (w97:T9)
            n95 = property on="Image Out" class="ImageControl"() -> ("ZoomInteger"=w95:cluster{"X":i32, "Y":i32})  [unwired: 2 in, 2 out]
            n96 = property on="Image Out" class="ImageControl"() -> ("ROI"=w101:T13)  [unwired: 2 in, 2 out]
            n97 = Unbundle By Name(w101) -> ("Contours"=w102:T14)
            n98 = local read "No Image\n File"() -> (w91:path)
            n99 = local read "Image File"() -> (w90:path)
            n100 = call "IMAQ Clear Overlay"("Image"=w97) -> ("Image Out"=w116:T9)  [unwired: 9 in, 1 out]
            n101 = Initialize Array(0) -> (w104:i32[])  [unwired: 1 in]
            n102 = Array Size(array=w102) -> (size(s)=w103:i32)
            n103 = Unbundle(w95) -> ("X"=w94:i32)  [unwired: 1 out]
            n104 = Equal?(x=w91, y=w90) -> (x = y?=w89:bool)
            n105 = local write "Zoom"(w94) -> ()
            n106 = Build Array(0.505025, 0.252522, 0.127742, 0.050345, 0.031129) -> (w111:dbl[])
            n107 = local read "Magnification"() -> (w112:u16)
            n108 = Array Subset(array=w111, index=w112, length=1) -> (w114:dbl[])
            n109 = case shown="True" w89 {
              tunnel: w92 -> [w153 _]
              frame False {
                n110 = local write "Image Center X"(w153) -> ()
              }
              frame True {
              }
            }
            n111 = To Double Precision Float(number=w114) -> (double precision float=w115:dbl[])
            n112 = for {
              N: w103 -> [_]
              shift-right: [w198] -> _
              shift-left: w102 -> [w198]
              shift-right: [w174] -> w99
              shift-left: w104 -> [w196]
              tunnel: w115 -> [w195]
              shift-right: [w192] -> _
              shift-left: w116 -> [w194]
              tunnel: w98 -> [w188]
              i -> [w191]
              n113 = Index Array(array=w198, index=w191) -> (element=w207:T20)
              n114 = Unbundle(w207) -> ("Points"=w206:i32[])  [unwired: 2 out]
              n115 = Array To Cluster(array=w206) -> (cluster=w205:T21)
              n116 = Unbundle(w205) -> ("Points[0]"=w187:i32, "Points[1]"=w184:i32, "Points[2]"=w197:i32, "Points[3]"=w203:i32)  [unwired: 5 out]
              n117 = Add(x=w187, y=10) -> (x+y=w185:i32)
              n118 = Subtract(x=w184, y=w203) -> (x-y=w202:i32)
              n119 = Subtract(x=w187, y=w197) -> (x-y=w204:i32)
              n120 = Square(x=w202) -> (x^2=w200:i32)
              n121 = Square(x=w204) -> (x^2=w201:i32)
              n122 = Add(x=w201, y=w200) -> (x+y=w199:i32)
              n123 = Square Root(x=w199) -> (sqrt(x)=w178:dbl)
              n124 = Multiply(x=w178, y=0.5) -> (x*y=w181:dbl)
              n125 = Add(x=w181, y=w184) -> (x+y=w183:dbl)
              n126 = Bundle(w185, w183) -> (w193:cluster{i32, dbl})  [unwired: 1 in]
              n127 = Multiply(x=w178, y=w195) -> (x*y=w177:dbl[])
              n128 = Index Array(array=w177) -> (element=w190:dbl)  [unwired: 1 in]
              n129 = Number To Fractional String(number=w190, precision (6)=0) -> (F-format string=w189:string)  [unwired: 2 in]
              n130 = call "IMAQ Overlay Text"("BG Color (Transparent)"=u32 0, "Text Color (black)"=u32 16448250, "Font, Size & Style"=w188, "String"=w189, "Origin"=w193, "Image"=w194) -> ("Image Out"=w192:T9)  [unwired: 4 in, 1 out]
              n131 = Build Array (concatenate)(w196, w177) -> (w175:dbl[])
              n132 = To Long Integer(number=w175) -> (32bit integer=w174:i32[])
            }
            n133 = local write "Distances"(w99) -> ()
            n134 = Add Array Elements(numeric array=w99) -> (sum=w100:i32)
            n135 = local write "Total Width"(w100) -> ()
          }
        }
        n136 = Unbundle By Name(w81) -> ("Manual-Temp"=w86:bool, "Manual-Width"=w85:bool, "Manuel-Length"=w84:bool, "Manuel-Dielectric"=w83:bool, "Manual Comments"=w82:bool)
        n137 = stacked-sequence {
          tunnel: w86 -> [w542 _ _]
          tunnel: w85 -> [_ w552 _]
          tunnel: w84 -> [_ _ w567]
          tunnel: w83 -> [_ _ w564]
          tunnel: w82 -> [_ _ w563]
          frame #0 {
            n138 = local read "Rec: Temp"() -> (w541:dbl)
            n139 = case shown="False" w542 {
              tunnel: w541 -> [w547 _]
              tunnel: [w544 w551] -> _
              frame False {
                n140 = local read "Rec: Temp"() -> (w545:dbl)
                n141 = property on="New: Temp" class="DigNum (strict)"("DisabledEnum"=1) -> ()  [unwired: 2 in, 2 out]
                n142 = Equal To 0?(x=w545) -> (x = 0?=w546:bool)
                n143 = local write "New: Temp"(w547) -> ()
                n144 = case shown="True" w546 {
                  tunnel: [w548 w549] -> w544
                  tunnel: w545 -> [w548 _]
                  frame False {
                  }
                  frame True {
                    n145 = local read "Room Temp"() -> (w549:dbl)
                  }
                }
                n146 = local write "New: Temp"(w544) -> ()
              }
              frame True {
                n147 = property on="New: Temp" class="DigNum (strict)"("DisabledEnum"=0) -> ()  [unwired: 2 in, 2 out]
                n148 = local read "New: Temp"() -> (w551:dbl)
              }
            }
          }
          frame #1 {
            n149 = case shown="False" w552 {
              frame False {
                n150 = property on="New: Width" class="DigNum (strict)"("DisabledEnum"=1) -> ()  [unwired: 2 in, 2 out]
              }
              frame True {
                (unwired) 0
              }
            }
            n151 = local read "Total Width"() -> (w558:dbl)
            n152 = Equal To 0?(x=w558) -> (x = 0?=w555:bool)
            n153 = local read "Rec: Width"() -> (w556:dbl)
            n154 = Not(x=w552) -> (.not. x?=w554:bool)
            n155 = Or(x=w555, y=w552) -> (x .or. y?=w557:bool)
            n156 = And(x=w555, y=w554) -> (x .and. y?=w553:bool)
            n157 = case shown="True" w553 {
              tunnel: w556 -> [_ w560]
              frame False {
              }
              frame True {
                n158 = local write "New: Width"(w560) -> ()
              }
            }
            n159 = case shown="True" w557 {
              tunnel: w558 -> [w561 _]
              frame False {
                n160 = local write "New: Width"(w561) -> ()
              }
              frame True {
                n161 = property on="New: Width" class="DigNum (strict)"("DisabledEnum"=0) -> ()  [unwired: 2 in, 2 out]
              }
            }
          }
          frame #2 {
            n162 = local read "Rec: Length"() -> (w568:dbl)
            n163 = case shown="False" w567 {
              tunnel: w568 -> [w576 _]
              frame False {
                n164 = local write "New: Length"(w576) -> ()
                n165 = property on="New: Length" class="DigNum (strict)"("DisabledEnum"=1) -> ()  [unwired: 2 in, 2 out]
              }
              frame True {
                n166 = property on="New: Length" class="DigNum (strict)"("DisabledEnum"=0) -> ()  [unwired: 2 in, 2 out]
              }
            }
            n167 = local read "Comments:"() -> (w565:string)
            n168 = local read "Rec: Dielectric (d)"() -> (w566:dbl)
            n169 = case shown="False" w563 {
              tunnel: w565 -> [w570 _]
              frame False {
                n170 = local write "New: Comments"(w570) -> ()
                n171 = property on="New: Comments" class="Str"("DisabledEnum"=1) -> ()  [unwired: 2 in, 2 out]
              }
              frame True {
                n172 = property on="New: Comments" class="Str"("DisabledEnum"=0) -> ()  [unwired: 2 in, 2 out]
              }
            }
            n173 = case shown="False" w564 {
              tunnel: w566 -> [w573 _]
              frame False {
                n174 = local write "New: Dielectric"(w573) -> ()
                n175 = property on="New: Dielectric" class="DigNum (strict)"("DisabledEnum"=1) -> ()  [unwired: 2 in, 2 out]
              }
              frame True {
                n176 = property on="New: Dielectric" class="DigNum (strict)"("DisabledEnum"=0) -> ()  [unwired: 2 in, 2 out]
              }
            }
          }
        }
        n177 = property on="Next File" class="Bool (strict)"("Value"=w67) -> (error out=w76:errorcluster)  [unwired: 2 in, 1 out]
        n178 = property on="Previous File" class="Bool (strict)"(error in=w76, "Value"=w67) -> (error out=w75:errorcluster)  [unwired: 1 in, 1 out]
        n179 = property on="Save" class="Bool (strict)"(error in=w75, "Value"=w67) -> (error out=w74:errorcluster)  [unwired: 1 in, 1 out]
        n180 = property on="Export" class="Bool (strict)"("Value"=w67) -> ()  [unwired: 2 in, 2 out]
        n181 = property on="Save Next" class="Bool (strict)"(error in=w74, "Value"=w67) -> (error out=w73:errorcluster)  [unwired: 1 in, 1 out]
        n182 = property on="Discard" class="Bool (strict)"(error in=w73, "Value"=w67) -> (error out=w72:errorcluster)  [unwired: 1 in, 1 out]
        n183 = property on="Save Lines" class="Bool (strict)"(error in=w72, "Value"=w67) -> ()  [unwired: 1 in, 2 out]
        n184 = property on="Close" class="Bool (strict)"("Value"=w67) -> ()  [unwired: 2 in, 2 out]
        n185 = Unbundle By Name(w77) -> ()  [unwired: 8 out]
        n186 = property on="Disable Flag" class="Bool (strict)"("Value"=w67) -> ()  [unwired: 2 in, 2 out]
        n187 = Cluster To Array(cluster=w77) -> (array=w87:bool[])
        n188 = call "Next State.vi"("Buttons []"=w87, "States []"=w88) -> ("Enum"=w80:T3)
        n189 = event shown="[12] \"Transfer File\": Value Change" {
          selector: _ -> [_ _ _ _ _ _ _ _ _ _ _ _ _]
          dyn-events: _ -> [_ _ _ _ _ _ _ _ _ _ _ _ _]
          timeout: 5 -> [_ _ _ _ _ _ _ _ _ _ _ _ _]
          tunnel: w80 -> [w427 _ _ _ _ _ _ _ _ _ _ _ _]
          tunnel: [w427 MegaAwesome_States."Re-Calculated Values" MegaAwesome_States."Re-Calculated Values" MegaAwesome_States."Re-Calculated Values" MegaAwesome_States."Re-Calculated Values" MegaAwesome_States."Calculated Values" MegaAwesome_States."Re-Calculated Values" MegaAwesome_States."Re-Calculated Values" MegaAwesome_States."Calculated Values" MegaAwesome_States."Re-Calculated Values" MegaAwesome_States."Re-Calculated Values" MegaAwesome_States."Read Data" MegaAwesome_States."Read Data"] -> w79
          tunnel: w70 -> [w426 w428 w430 w432 w434 w436 w438 w463 w488 w490 w511 _ w539]
          tunnel: [w426 w428 w430 w432 w434 w436 w438 w463 w488 w490 w511 w530 w539] -> w69
          tunnel: w68 -> [_ _ _ _ _ _ _ _ _ _ _ w529 _]
          event Timeout {
            n190 = event-data() -> ()  [unwired: 1 in, 2 out]
          }
          event "New: Dielectric": Value Change {
            n191 = event-data() -> ()  [unwired: 1 in, 5 out]
          }
          event "New: Length": Value Change {
            n192 = event-data() -> ()  [unwired: 1 in, 5 out]
          }
          event "New: Width": Value Change {
            n193 = event-data() -> ()  [unwired: 1 in, 5 out]
          }
          event "New: Temp": Value Change {
            n194 = event-data() -> ()  [unwired: 1 in, 5 out]
          }
          event "Num Pts Log", "Transport Style Controls", "Num Pts": Value Change {
            n195 = event-data() -> ()  [unwired: 1 in, 5 out]
          }
          event "Sat-Trans Slider": Value Change {
            n196 = event-data() -> ()  [unwired: 1 in, 5 out]
            n197 = local read "Sqrt-Sat"() -> (w462:cluster{dbl[], dbl[]}[])
            n198 = Decimate 1D Array(w462) -> (w446:cluster{dbl[], dbl[]}[], w447:cluster{dbl[], dbl[]}[])
            n199 = local read "Slider Min"() -> (w443:dbl)
            n200 = local read "Sat-Trans Slider"() -> (w441:dbl)
            n201 = Array To Cluster(array=w446) -> (cluster=w461:T22)
            n202 = local read "New: Dielectric"() -> (w456:dbl)
            n203 = local read "Num Pts"() -> (w439:dbl)
            n204 = local read "New: Width"() -> (w458:dbl)
            n205 = local read "New: Length"() -> (w457:dbl)
            n206 = Unbundle(w461) -> ("[0]"=w460:cluster{dbl[], dbl[]})  [unwired: 8 out]
            n207 = Absolute Value(x=w443) -> (abs(x)=w442:dbl)
            n208 = Unbundle(w460) -> (w444:dbl[], w459:dbl[])
            n209 = Add(x=w441, y=w442) -> (x+y=w440:dbl)
            n210 = Array Subset(array=w444, index=w440, length=w439) -> (w454:dbl[])
            n211 = local write "Sat Vg Array-Used"(w454) -> ()
            n212 = Array Subset(array=w459, index=w440, length=w439) -> (w455:dbl[])
            n213 = call "Mobility-Vt-Used Pts_Saturation.vi"("Width"=w458, "Length"=w457, "Dielectric (d)"=w456, "Sat Id Used"=w455, "Vg Used"=w454) -> ("Vt"=w450:dbl, "Mobility"=w451:dbl)  [unwired: 4 in, 1 out]
            n214 = local write "Index-Sat"(w440) -> ()
            n215 = local write "Sat Id-Used"(w455) -> ()
            n216 = Bundle(w454, w455) -> (w448:cluster{dbl[], dbl[]})  [unwired: 1 in]
            n217 = local read "Re-Calculated Values Cluster"() -> (w453:T10)
            n218 = Bundle By Name(cluster=w453, "Mobility-Sat"=w451, "Vt-Sat"=w450) -> (w452:T10)
            n219 = local write "Re-Calculated Values Cluster"(w452) -> ()
            n220 = Build Array (concatenate)(w446, w447, w448) -> (w445:cluster{dbl[], dbl[]}[])
            n221 = local write "Sqrt-Sat"(w445) -> ()
          }
          event "Lin-Trans Slider": Value Change {
            n222 = event-data() -> ()  [unwired: 1 in, 5 out]
            n223 = local read "Sqrt-Lin"() -> (w487:cluster{dbl[], dbl[]}[])
            n224 = Decimate 1D Array(w487) -> (w472:cluster{dbl[], dbl[]}[], w473:cluster{dbl[], dbl[]}[])
            n225 = local read "Slider Min"() -> (w469:dbl)
            n226 = Array To Cluster(array=w472) -> (cluster=w486:T22)
            n227 = local read "Lin-Trans Slider"() -> (w467:dbl)
            n228 = local read "New: Dielectric"() -> (w480:dbl)
            n229 = local read "Num Pts"() -> (w483:dbl)
            n230 = local read "New: Width"() -> (w482:dbl)
            n231 = local read "New: Length"() -> (w481:dbl)
            n232 = local read "Lin Vd"() -> (w464:dbl)
            n233 = Unbundle(w486) -> ("[0]"=w485:cluster{dbl[], dbl[]})  [unwired: 8 out]
            n234 = Absolute Value(x=w469) -> (abs(x)=w468:dbl)
            n235 = Unbundle(w485) -> (w470:dbl[], w484:dbl[])
            n236 = Add(x=w467, y=w468) -> (x+y=w466:dbl)
            n237 = Array Subset(array=w470, index=w466, length=w483) -> (w478:dbl[])
            n238 = local write "Lin-Vg Array-Used"(w478) -> ()
            n239 = Array Subset(array=w484, index=w466, length=w483) -> (w479:dbl[])
            n240 = call "Mobility-Vt-Used Pts_Linear.vi"("Width"=w482, "Length"=w481, "Vd"=w464, "Dielectric (d)"=w480, "Id Used"=w479, "Vg Used"=w478) -> ("Mobility"=w475:dbl)  [unwired: 3 in, 2 out]
            n241 = local write "Index-Lin"(w466) -> ()
            n242 = local write "Lin Id-Used"(w479) -> ()
            n243 = Bundle(w478, w479) -> (w474:cluster{dbl[], dbl[]})  [unwired: 1 in]
            n244 = local read "Re-Calculated Values Cluster"() -> (w477:T10)
            n245 = Bundle By Name(cluster=w477, "Moblitity-Lin"=w475) -> (w476:T10)
            n246 = local write "Re-Calculated Values Cluster"(w476) -> ()
            n247 = Build Array (concatenate)(w472, w473, w474) -> (w471:cluster{dbl[], dbl[]}[])
            n248 = local write "Sqrt-Lin"(w471) -> ()
          }
          event "Image Analysis", "1) Transport": Value Change {
            n249 = event-data() -> ()  [unwired: 1 in, 5 out]
          }
          event "Sat-Log Slider": Value Change {
            n250 = event-data() -> ()  [unwired: 1 in, 5 out]
            n251 = local read "Sat-Log"() -> (w493:cluster{dbl[], dbl[]}[])
            n252 = Decimate 1D Array(w493) -> (w500:cluster{dbl[], dbl[]}[], w501:cluster{dbl[], dbl[]}[])
            n253 = local read "Slider Min"() -> (w497:dbl)
            n254 = Array To Cluster(array=w500) -> (cluster=w510:T22)
            n255 = local read "Num Pts Log"() -> (w507:dbl)
            n256 = local read "Sat-Log Slider"() -> (w495:dbl)
            n257 = Unbundle(w510) -> ("[0]"=w509:cluster{dbl[], dbl[]})  [unwired: 8 out]
            n258 = Absolute Value(x=w497) -> (abs(x)=w496:dbl)
            n259 = Unbundle(w509) -> (w498:dbl[], w508:dbl[])
            n260 = Add(x=w495, y=w496) -> (x+y=w492:dbl)
            n261 = Array Subset(array=w498, index=w492, length=w507) -> (w505:dbl[])
            n262 = Array Subset(array=w508, index=w492, length=w507) -> (w506:dbl[])
            n263 = local write "Vg Array-Log-Used"(w505) -> ()
            n264 = local write "IndexLog-Sat"(w492) -> ()
            n265 = Bundle(w505, w506) -> (w491:cluster{dbl[], dbl[]})  [unwired: 1 in]
            n266 = call "STS-Used.vi"("Id Used"=w506, "Vg-Used"=w505) -> ("STS"=w502:dbl)  [unwired: 9 in]
            n267 = local write "Sat Id-Log-Used"(w506) -> ()
            n268 = local read "Re-Calculated Values Cluster"() -> (w504:T10)
            n269 = Bundle By Name(cluster=w504, "STS"=w502) -> (w503:T10)
            n270 = local write "Re-Calculated Values Cluster"(w503) -> ()
            n271 = Build Array (concatenate)(w500, w501, w491) -> (w499:cluster{dbl[], dbl[]}[])
            n272 = local write "Sat-Log"(w499) -> ()
          }
          event "Lin-Log Slider": Value Change {
            # "No Indicator for Lin-Log Slider Use"
            n273 = event-data() -> ()  [unwired: 1 in, 5 out]
            n274 = local read "Log-Lin"() -> (w515:cluster{dbl[], dbl[]}[])
            n275 = Decimate 1D Array(w515) -> (w521:cluster{dbl[], dbl[]}[], w522:cluster{dbl[], dbl[]}[])
            n276 = local read "Slider Min"() -> (w518:dbl)
            n277 = Array To Cluster(array=w521) -> (cluster=w528:T22)
            n278 = local read "Num Pts Log"() -> (w525:dbl)
            n279 = local read "Lin-Log Slider"() -> (w516:dbl)
            n280 = Unbundle(w528) -> ("[0]"=w527:cluster{dbl[], dbl[]})  [unwired: 8 out]
            n281 = Absolute Value(x=w518) -> (abs(x)=w517:dbl)
            n282 = Unbundle(w527) -> (w519:dbl[], w526:dbl[])
            n283 = Add(x=w516, y=w517) -> (x+y=w514:dbl)
            n284 = Array Subset(array=w519, index=w514, length=w525) -> (w523:dbl[])
            n285 = local write "Lin-Vg Array-Log Used"(w523) -> ()
            n286 = Array Subset(array=w526, index=w514, length=w525) -> (w524:dbl[])
            n287 = local write "IndexLog-Sat"(w514) -> ()
            n288 = Bundle(w523, w524) -> (w513:cluster{dbl[], dbl[]})  [unwired: 1 in]
            n289 = call "STS-Used.vi"("Id Used"=w524, "Vg-Used"=w523) -> ()  [unwired: 9 in, 1 out]
            n290 = local write "Lin Id-Log Used"(w524) -> ()
            n291 = Build Array (concatenate)(w521, w522, w513) -> (w520:cluster{dbl[], dbl[]}[])
            n292 = local write "Log-Lin"(w520) -> ()
          }
          event "Index Array": Value Change {
            n293 = event-data() -> ()  [unwired: 1 in, 5 out]
            n294 = Strip Path(path=w529) -> (stripped path=w535:path)  [unwired: 1 out]
            n295 = local write "Transfer Folder"(w535) -> ()
            n296 = List Folder(path=w535) -> (filenames=w531:string[])  [unwired: 3 in, 3 out]
            n297 = local read "Index Array"() -> (w530:u16)
            n298 = Path To String(path=w535) -> (string=w536:string)
            n299 = Index Array(array=w531, index=w530) -> (element=w537:string)
            n300 = Concatenate Strings(w536, "\\", w537) -> (w533:string)
            n301 = String To Path(string=w533) -> (path=w532:path)
            n302 = local write "Transfer File"(w532) -> ()
          }
          event "Transfer File": Value Change {
            n303 = event-data() -> ()  [unwired: 1 in, 5 out]
          }
        }
      }
      frame "Read Data" {
        n304 = call "IMAQ Dispose"("All Images? (No)"=TRUE) -> ()  [unwired: 5 in, 1 out]
        n305 = case shown="False" "Disable Flag" {
          tunnel: w581 -> [_ w611]
          tunnel: [w607 w608] -> w580
          tunnel: w578 -> [w607 _]
          frame False {
          }
          frame True {
            n306 = local read "Transfer Folder"() -> (w610:path)
            n307 = List Folder(path=w610) -> (filenames=w612:string[])  [unwired: 3 in, 3 out]
            n308 = Index Array(array=w612, index=w611) -> (element=w609:string)
            n309 = Build Path(base path=w610, name or relative path=w609) -> (appended path=w608:path)
            n310 = local write "Transfer File"(w608) -> ()
          }
        }
        n311 = call "Recorded Values.vi"("Path"=w580) -> ("Recorded Char"=w606:T10, "Recorded Prop"=w596:T2, "Fabrication Prop"=w593:T5)  [unwired: 8 in]
        n312 = Strip Path(path=w580) -> (stripped path=w592:path, name=w591:string)
        n313 = local write "Fabrication Prop"(w593) -> ()
        n314 = local write "Recorded Prop"(w596) -> ()
        n315 = Unbundle By Name(w596) -> ("Date Recorded"=w595:string, "Index"=w594:string, "Length"=w587:dbl, "Width"=w586:dbl, "Sample Temp"=w585:dbl)
        n316 = local write "Recorded Values Cluster"(w606) -> ()
        n317 = Unbundle By Name(w596) -> ("Sample Temp"=w599:dbl)
        n318 = Unbundle By Name(w593) -> ("Dielectric (nm)"=w588:dbl, "Comments"=w589:string)
        n319 = List Folder(path=w592) -> (filenames=w584:string[])  [unwired: 3 in, 3 out]
        n320 = local write "Rec: Dielectric (d)"(w588) -> ()
        n321 = local write "Date Created"(w595) -> ()
        n322 = local write "Index"(w594) -> ()
        n323 = local write "Rec: Length"(w587) -> ()
        n324 = local write "Rec: Width"(w586) -> ()
        n325 = local write "Rec: Temp"(w585) -> ()
        n326 = Equal To 0?(x=w599) -> (x = 0?=w602:bool)
        n327 = Number To Decimal String(number=w599) -> (decimal integer string=w603:string)  [unwired: 1 in]
        n328 = local write "Comments:"(w589) -> ()
        n329 = Search 1D Array(1D array=w584, element=w591) -> (index of element=w583:i32)  [unwired: 1 in]
        n330 = Equal?(x="", y=w603) -> (x = y?=w601:bool)
        n331 = Index Array(array=w584, index=w583) -> (element=w590:string)
        n332 = local write "New: Width"(w586) -> ()
        n333 = local write "New: Length"(w587) -> ()
        n334 = local write "New: Temp"(w585) -> ()
        n335 = local write "Index Array"(w583) -> ()
        n336 = Or(x=w602, y=w601) -> (x .or. y?=w600:bool)
        n337 = local write "New: Dielectric"(w588) -> ()
        n338 = local write "Data Name:"(w590) -> ()
        n339 = case shown="False" w600 {
          tunnel: [w613 w614] -> w597
          tunnel: w599 -> [w613 _]
          frame False {
          }
          frame True {
            n340 = local read "Room Temp"() -> (w614:dbl)
          }
        }
        n341 = local write "New: Temp"(w597) -> ()
        n342 = Bundle By Name(cluster=w596, "Sample Temp"=w597) -> (w598:T2)
        n343 = local write "Recorded Prop"(w598) -> ()
      }
      frame "Calculated Values" {
        n344 = case shown="True" w618 {
          selector: w618 -> [w692 _]
          tunnel: w628 -> [w691 w703]
          tunnel: w616 -> [w690 w699]
          tunnel: w615 -> [w695 w697]
          frame False {
            n345 = call "TRF to TSP Plot_09_21_12a_JW.vi"("Plot Transport"=w692, "No Transport File"=w695, "Transport Folder"=w690, "Transfer File"=w691) -> ("Transport"=w693:cluster{ext[], ext[]}[], "Transport File"=w694:path, "Transport Name"=w689:string)  [unwired: 5 in]
            n346 = local write "Transport"(w693) -> ()
            n347 = local write "Transport\nFile"(w694) -> ()
            n348 = local write "Transport Name:"(w689) -> ()
          }
          frame True {
            n349 = local read "Transport Style Controls"() -> (w702:T11)
            n350 = call "TRF to TSP Plot_09_21_12a_JW.vi"("Transport Graph Properties"=w702, "No Transport File"=w697, "Transport Folder"=w699, "Transfer File"=w703) -> ("Transport"=w701:cluster{ext[], ext[]}[], "Transport File"=w698:path, "Transport Name"=w696:string)  [unwired: 5 in]
            n351 = Array Size(array=w701) -> (size(s)=w700:i32)
            n352 = local write "Transport"(w701) -> ()
            n353 = for {
              N: w700 -> [_]
              tunnel: w702 -> [w707]
              i -> [w706]
              n354 = Unbundle By Name(w707) -> ("Transport Line Size"=w704:u16, "Transport Line Color"=w705:u32)
              n355 = property on="Transport" class="XYGraph (strict)"("Active Plot"=w706, "Plot.Plot Color"=w705, "Plot.Line Width"=w704) -> ()  [unwired: 2 in, 2 out]
            }
            n356 = local write "Transport\nFile"(w698) -> ()
            n357 = local write "Transport Name:"(w696) -> ()
          }
        }
        n358 = case shown="True" w617 {
          tunnel: w648 -> [_ w677]
          tunnel: w647 -> [w669 w683]
          tunnel: w628 -> [_ w682]
          frame False {
            n359 = call "Vision Acquisition2"("Image Path"=w669) -> ("Image Out"=w668:T9)  [unwired: 25 in, 1 out]
            n360 = local write "Image Out"(w668) -> ()
            n361 = local write "Image Preview"(w668) -> ()
          }
          frame True {
            n362 = local read "Image Center X"() -> (w670:i32)
            n363 = call "Image from TRF Display.vi"("Image Center X"=w670, "No Image File"=w683, "Image Folder"=w677, "Transfer File"=w682) -> ("Image Preview"=w678:T9, "Image Out"=w679:T9, "Image File"=w680:path, "Image Name"=w681:string, "ROI File"=w674:path)  [unwired: 3 in]
            n364 = invoke on="Image Out" class="ImageControl" method="Clear ROI"() -> ()  [unwired: 3 in, 3 out]
            n365 = local write "Image File"(w680) -> ()
            n366 = local write "Image Name"(w681) -> ()
            n367 = local write "Image Out"(w679) -> ()
            n368 = local write "Image Preview"(w678) -> ()
            n369 = call <vilib>:"Check if File or Folder Exists.vi"("path"=w674) -> ("file or folder exists?"=w675:bool, "dup path"=w676:path)  [unwired: 8 in, 1 out]
            n370 = case shown="True" w675 {
              tunnel: w676 -> [_ w684]
              frame False {
              }
              frame True {
                n371 = Read from Text File(file (use dialog)=w684) -> (text=w688:string)  [unwired: 3 in, 3 out]
                n372 = property on="Image Out" class="ImageControl"() -> ("ROI"=w685:T13)  [unwired: 2 in, 2 out]
                n373 = Unflatten From String(type=w685, binary string=w688) -> (value=w686:T13, error out=w687:errorcluster)  [unwired: 3 in, 1 out]
                n374 = property on="Image Out" class="ImageControl"(error in=w687, "ROI"=w686) -> ()  [unwired: 1 in, 2 out]
              }
            }
            n375 = local read "Image Center X"() -> (w671:i32)
            n376 = Bundle("Image Center X"=w671, 0) -> (w673:cluster{"Image Center X":i32, i32})  [unwired: 1 in]
            n377 = property on="Image Out" class="ImageControl"("Image Center Position"=w673) -> ()  [unwired: 2 in, 2 out]
          }
        }
        n378 = local read "Fabrication Prop"() -> (w657:T5)
        n379 = local read "Recorded Prop"() -> (w650:T2)
        n380 = local read "Calculated Values Cluster"() -> (w667:T10)
        n381 = call "Mobility-Vt Calculator-File.vi"("NumPts"=w652, "Path"=w628) -> ("Used Points"=w645:T23, "Graph Cluster"=w634:T24, "Lin Vd"=w641:dbl, "Output"=w665:T25)  [unwired: 6 in]
        n382 = call "STS Calculator-File.vi"("NumPts"=w651, "Path"=w628) -> ("Used Points"=w639:T26, "XY Graph-Sat"=w621:cluster{dbl[], dbl[]}[], "XY Graph-Lin"=w622:cluster{dbl[], dbl[]}[], "Ouput"=w660:cluster{"STS-Sat":dbl, "STS-Lin":dbl})  [unwired: 6 in]
        n383 = Unbundle By Name(w657) -> ("Dielectric (nm)"=w655:dbl)
        n384 = Unbundle By Name(w650) -> ("Sample Temp"=w649:dbl)
        n385 = Unbundle By Name(w665) -> ("Mobility-Sat"=w664:dbl, "Vt-Sat"=w656:dbl, "Mobility-Lin"=w663:dbl, "Off I-Sat"=w662:dbl, "On/Off I-Sat"=w661:dbl)  [unwired: 1 out]
        n386 = local write "Lin Vd"(w641) -> ()
        n387 = Unbundle By Name(w660) -> ("STS-Sat"=w654:dbl)  [unwired: 1 out]
        n388 = local write "Sat-Log"(w621) -> ()
        n389 = local write "Log-Lin"(w622) -> ()
        n390 = call "Trap Density_VT.vi"("VT"=w656, "Dielectric"=w655) -> ("Trap Density-VT"=w659:dbl)
        n391 = call "Trap Density_STS.vi"("Temp (T) [K]"=w649, "S.T.S. (S)"=w654, "Dielectric"=w655) -> ("Trap Density (N)"=w658:dbl)  [unwired: 8 in]
        n392 = Bundle By Name(cluster=w667, "Mobility-Sat"=w664, "Moblitity-Lin"=w663, "On/Off"=w661, "Off Current"=w662, "Vt-Sat"=w656, "STS"=w654, "Trap Density-VT"=w659, "Trap Density-STS"=w658) -> (w666:T10)
        n393 = Unbundle By Name(w639) -> ("Sat Vg Used"=w638:dbl[], "Sat Log(Id) Used"=w637:dbl[], "Lin Vg Used"=w636:dbl[], "Lin Log(Id) Used"=w635:dbl[], "STS Index-Sat"=w619:dbl, "STS Index-Lin"=w620:dbl)
        n394 = Unbundle By Name(w645) -> ("Sat Vg Used"=w644:dbl[], "Sat Sqrt(Id) Used"=w643:dbl[], "Lin Vg Used"=w642:dbl[], "Lin Sqrt(Id) Used"=w640:dbl[], "Index-Lin"=w630:dbl, "Index-Sat"=w629:dbl)
        n395 = local write "Vg Array-Log-Used"(w638) -> ()
        n396 = local write "Sat Id-Log-Used"(w637) -> ()
        n397 = local write "Lin-Vg Array-Log Used"(w636) -> ()
        n398 = local write "Lin Id-Log Used"(w635) -> ()
        n399 = local write "IndexLog-Sat"(w619) -> ()
        n400 = local write "Index-Lin"(w620) -> ()
        n401 = local write "Calculated Values Cluster"(w666) -> ()
        n402 = local write "Sat Vg Array-Used"(w644) -> ()
        n403 = local write "Sat Id-Used"(w643) -> ()
        n404 = local write "Lin-Vg Array-Used"(w642) -> ()
        n405 = local write "Lin Id-Used"(w640) -> ()
        n406 = local write "Index-Sat"(w629) -> ()
        n407 = local write "Index-Lin"(w630) -> ()
        n408 = local write "Lin-Log Slider"(w620) -> ()
        n409 = local write "Sat-Log Slider"(w619) -> ()
        n410 = local write "Sat-Trans Slider"(w629) -> ()
        n411 = local write "Lin-Trans Slider"(w630) -> ()
        n412 = Unbundle By Name(w634) -> ("Raw Sat"=w627:cluster{dbl[], dbl[]}[], "Sqrt Sat"=w631:cluster{dbl[], dbl[]}[], "Raw Lin"=w633:cluster{dbl[], dbl[]}[], "Sqrt Lin"=w632:cluster{dbl[], dbl[]}[])
        n413 = Index Array(array=w627) -> (element=w626:cluster{dbl[], dbl[]})  [unwired: 1 in]
        n414 = Unbundle(w626) -> (w625:dbl[])  [unwired: 1 out]
        n415 = Array Max & Min(array=w625) -> (max value=w624:dbl, min value=w623:dbl)  [unwired: 2 out]
        n416 = property on="Sat-Trans Slider" class="Slide (strict)"("Scale.Maximum"=w624, "Scale.Minimum"=w623) -> ()  [unwired: 2 in, 2 out]
        n417 = property on="Lin-Trans Slider" class="Slide (strict)"("Scale.Maximum"=w624, "Scale.Minimum"=w623) -> ()  [unwired: 2 in, 2 out]
        n418 = property on="Sat-Log Slider" class="Slide (strict)"("Scale.Maximum"=w624, "Scale.Minimum"=w623) -> ()  [unwired: 2 in, 2 out]
        n419 = property on="Lin-Log Slider" class="Slide (strict)"("Scale.Maximum"=w624, "Scale.Minimum"=w623) -> ()  [unwired: 2 in, 2 out]
        n420 = local write "Slider Max"(w624) -> ()
        n421 = local write "Slider Min"(w623) -> ()
        n422 = local write "Raw- Sat"(w627) -> ()
        n423 = local write "Raw- Lin"(w633) -> ()
        n424 = local write "Sqrt-Sat"(w631) -> ()
        n425 = local write "Sqrt-Lin"(w632) -> ()
      }
      frame "Re-Calculated Values" {
        n426 = local read "Vg Array-Log-Used"() -> (w716:dbl[])
        n427 = local read "Sat Vg Array-Used"() -> (w724:dbl[])
        n428 = local read "Lin-Vg Array-Used"() -> (w730:dbl[])
        n429 = local read "Sat Id-Log-Used"() -> (w715:dbl[])
        n430 = local read "New: Dielectric"() -> (w728:dbl)
        n431 = local read "New: Dielectric"() -> (w713:dbl)
        n432 = local read "New: Length"() -> (w727:dbl)
        n433 = local read "New: Length"() -> (w723:dbl)
        n434 = local read "New: Width"() -> (w726:dbl)
        n435 = local read "New: Width"() -> (w722:dbl)
        n436 = local read "Lin Id-Used"() -> (w729:dbl[])
        n437 = local read "Sat Id-Used"() -> (w721:dbl[])
        n438 = local read "Re-Calculated Values Cluster"() -> (w732:T10)
        n439 = local read "New: Dielectric"() -> (w712:dbl)
        n440 = local read "New: Temp"() -> (w711:dbl)
        n441 = local read "Lin Vd"() -> (w708:dbl)
        n442 = call "Mobility-Vt-Used Pts_Saturation.vi"("Width"=w722, "Length"=w723, "Dielectric (d)"=w713, "Sat Id Used"=w721, "Vg Used"=w724) -> ("Vt"=w719:dbl, "Mobility"=w720:dbl)  [unwired: 4 in, 1 out]
        n443 = call "STS-Used.vi"("Id Used"=w715, "Vg-Used"=w716) -> ("STS"=w714:dbl)  [unwired: 9 in]
        n444 = call "Mobility-Vt-Used Pts_Linear.vi"("Width"=w726, "Length"=w727, "Vd"=w708, "Dielectric (d)"=w728, "Id Used"=w729, "Vg Used"=w730) -> ("Mobility"=w725:dbl)  [unwired: 3 in, 2 out]
        n445 = call "Trap Density_VT.vi"("VT"=w719, "Dielectric"=w713) -> ("Trap Density-VT"=w718:dbl)
        n446 = call "Trap Density_STS.vi"("Temp (T) [K]"=w711, "S.T.S. (S)"=w714, "Dielectric"=w712) -> ("Trap Density (N)"=w710:dbl)  [unwired: 8 in]
        n447 = Bundle By Name(cluster=w732, "Mobility-Sat"=w720, "Moblitity-Lin"=w725, "Vt-Sat"=w719, "STS"=w714, "Trap Density-VT"=w718, "Trap Density-STS"=w710) -> (w731:T10)
        n448 = local write "Re-Calculated Values Cluster"(w731) -> ()
      }
      frame "Next File" {
        n449 = call "IMAQ Dispose"("All Images? (No)"=TRUE) -> ()  [unwired: 5 in, 1 out]
        n450 = Strip Path(path=w750) -> (stripped path=w740:path, name=w748:string)
        n451 = local write "Transfer Folder"(w740) -> ()
        n452 = List Folder(path=w740) -> (filenames=w734:string[], error out=w743:errorcluster)  [unwired: 3 in, 2 out]
        n453 = Array Size(array=w734) -> (size(s)=w747:i32)
        n454 = Search 1D Array(1D array=w734, element=w748) -> (index of element=w745:i32)  [unwired: 1 in]
        n455 = Decrement(x=w747) -> (x-1=w746:i32)
        n456 = Equal?(x=w746, y=w745) -> (x = y?=w744:bool)
        n457 = case shown="False" w744 {
          tunnel: w736 -> [w753 _]
          tunnel: [w752 0] -> w735
          tunnel: w743 -> [w751 w754]
          tunnel: [w751 w754] -> _
          frame False {
            n458 = Increment(x=w753) -> (x+1=w752:i32)
          }
          frame True {
          }
        }
        n459 = Path To String(path=w740) -> (string=w741:string)
        n460 = Index Array(array=w734, index=w735) -> (element=w742:string)
        n461 = Concatenate Strings(w741, "\\", w742) -> (w738:string)
        n462 = String To Path(string=w738) -> (path=w737:path)
        n463 = local write "Transfer File"(w737) -> ()
      }
      frame "Previous File" {
        n464 = call "IMAQ Dispose"("All Images? (No)"=TRUE) -> ()  [unwired: 5 in, 1 out]
        n465 = Strip Path(path=w763) -> (stripped path=w760:path, name=w772:string)
        n466 = local write "Transfer Folder"(w760) -> ()
        n467 = List Folder(path=w760) -> (filenames=w764:string[], error out=w769:errorcluster)  [unwired: 3 in, 2 out]
        n468 = Array Size(array=w764) -> (size(s)=w758:i32)
        n469 = Search 1D Array(1D array=w764, element=w772) -> (index of element=w771:i32)  [unwired: 1 in]
        n470 = Decrement(x=w758) -> (x-1=w757:i32)
        n471 = Equal To 0?(x=w771) -> (x = 0?=w770:bool)
        n472 = case shown="False" w770 {
          tunnel: w762 -> [w776 _]
          tunnel: [w775 w777] -> w761
          tunnel: w769 -> [w774 w778]
          tunnel: [w774 w778] -> _
          tunnel: w757 -> [_ w777]
          frame False {
            n473 = Decrement(x=w776) -> (x-1=w775:i32)
          }
          frame True {
          }
        }
        n474 = Path To String(path=w760) -> (string=w759:string)
        n475 = Index Array(array=w764, index=w761) -> (element=w768:string)
        n476 = Concatenate Strings(w759, "\\", w768) -> (w766:string)
        n477 = String To Path(string=w766) -> (path=w765:path)
        n478 = local write "Transfer File"(w765) -> ()
      }
      frame "Discard File" {
        n479 = flat-sequence {
          tunnel: w784 -> [w787]
          tunnel: [w787] -> w783
          tunnel: [w786] -> w780
          tunnel: w783 -> [w799]
          tunnel: w780 -> [w792]
          tunnel: [w791] -> w779
          frame #0 {
            n480 = Strip Path(path=w787) -> (stripped path=w790:path, name=w789:string)
            n481 = List Folder(path=w790) -> (filenames=w788:string[])  [unwired: 3 in, 3 out]
            n482 = Search 1D Array(1D array=w788, element=w789) -> (index of element=w786:i32)  [unwired: 1 in]
          }
          frame #1 {
            n483 = Strip Path(path=w799) -> (stripped path=w800:path, name=w798:string)
            n484 = String Subset(string=w798, offset (0)=0, length (rest)=1) -> (substring=w795:string)
            n485 = Equal?(x=w795, y="X") -> (x = y?=w793:bool)
            n486 = case shown="True" w793 {
              tunnel: w800 -> [w807 _]
              tunnel: w799 -> [w803 _]
              tunnel: w798 -> [w802 _]
              tunnel: w792 -> [w801 w811]
              tunnel: [w801 w810] -> w791
              frame False {
                n487 = Path To String(path=w807) -> (string=w806:string)
                n488 = Concatenate Strings(w806, "\\", "X_", w802) -> (w805:string)
                n489 = String To Path(string=w805) -> (path=w804:path)
                n490 = Move(source path=w803, 10:w804) -> ()  [unwired: 3 in, 3 out]
              }
              frame True {
                n491 = Increment(x=w811) -> (x+1=w810:i32)
              }
            }
          }
        }
        n492 = property on="Disable Flag" class="Bool (strict)"("Value"=TRUE) -> ()  [unwired: 2 in, 2 out]
        n493 = call "IMAQ Dispose"("All Images? (No)"=TRUE) -> ()  [unwired: 5 in, 1 out]
      }
      frame "Save" {
        n494 = stacked-sequence {
          seq-local: [w827 _] -> [_ w1324]
          seq-local: [w826 _] -> [_ w1322]
          tunnel: w818 -> [w828 w1325]
          frame #0 {
            # "Saves each Re-calculated parameter in sequence"
            n495 = stacked-sequence {
              tunnel: [_ _ _ _ _ _ _ _ _ _ _ _ _ w1292] -> w826
              tunnel: w828 -> [w848 _ _ _ _ _ _ _ _ _ _ _ _ _]
              frame #0 {
                n496 = call-poly <vilib>:"Read From Spreadsheet File.vi"("file path (dialog if empty)"=w848) -> ("all rows"=w847:string[][])  [unwired: 6 in, 4 out]
                n497 = Array Size(array=w847) -> (size(s)=w852:i32[])
                n498 = Array Subset(array=w847, index (row)=0, index (col)=0, length (col)=3) -> (w856:string[][])  [unwired: 1 in]
                n499 = Index Array(array=w852, index=0) -> (element=w850:i32)
                n500 = Reshape Array(w856, w850) -> (w849:string[])
                n501 = Search 1D Array(1D array=w849, element="Dielectric (nm):") -> (index of element=w859:i32)  [unwired: 1 in]
                n502 = Equal?(x=w859, y=-1) -> (x = y?=w858:bool)
                n503 = case shown="False" w858 {
                  tunnel: w847 -> [w867 w871]
                  tunnel: w859 -> [w863 _]
                  tunnel: [w862 w871] -> w857
                  frame False {
                    n504 = local read "Rec: Dielectric (d)"() -> (w869:dbl)
                    n505 = Number To Fractional String(number=w869) -> (F-format string=w864:string)  [unwired: 3 in]
                    n506 = Divide(x=w863, y=3) -> (x/y=w866:dbl)
                    n507 = To Word Integer(number=w866) -> (16bit integer=w865:i16)
                    n508 = Replace Array Subset(array=w867, new element=w864, index (row)=w865, index (col)=1) -> (w862:string[][])
                  }
                  frame True {
                  }
                }
                n509 = local write "Save Array"(w857) -> ()
              }
              frame #1 {
                n510 = local read "Save Array"() -> (w873:string[][])
                n511 = Array Size(array=w873) -> (size(s)=w876:i32[])
                n512 = Array Subset(array=w873, index (row)=0, index (col)=0, length (col)=3) -> (w880:string[][])  [unwired: 1 in]
                n513 = Index Array(array=w876, index=0) -> (element=w874:i32)
                n514 = Reshape Array(w880, w874) -> (w872:string[])
                n515 = Search 1D Array(1D array=w872, element="Comments:") -> (index of element=w883:i32)  [unwired: 1 in]
                n516 = Equal?(x=w883, y=-1) -> (x = y?=w882:bool)
                n517 = case shown="False" w882 {
                  tunnel: w873 -> [w891 w894]
                  tunnel: w883 -> [w888 _]
                  tunnel: [w887 w894] -> w881
                  frame False {
                    n518 = local read "New: Comments"() -> (w886:string)
                    n519 = Divide(x=w888, y=3) -> (x/y=w890:dbl)
                    n520 = To Word Integer(number=w890) -> (16bit integer=w889:i16)
                    n521 = Replace Array Subset(array=w891, new element=w886, index (row)=w889, index (col)=1) -> (w887:string[][])
                  }
                  frame True {
                  }
                }
                n522 = local write "Save Array"(w881) -> ()
              }
              frame #2 {
                n523 = local read "Save Array"() -> (w896:string[][])
                n524 = Array Size(array=w896) -> (size(s)=w899:i32[])
                n525 = Array Subset(array=w896, index (row)=0, index (col)=0, length (col)=3) -> (w903:string[][])  [unwired: 1 in]
                n526 = Index Array(array=w899, index=0) -> (element=w897:i32)
                n527 = Reshape Array(w903, w897) -> (w895:string[])
                n528 = Search 1D Array(1D array=w895, element="Length (um):") -> (index of element=w906:i32)  [unwired: 1 in]
                n529 = Equal?(x=w906, y=-1) -> (x = y?=w905:bool)
                n530 = case shown="False" w905 {
                  tunnel: w896 -> [w916 w919]
                  tunnel: w906 -> [w913 _]
                  tunnel: [w912 w919] -> w904
                  frame False {
                    n531 = local read "New: Length"() -> (w909:dbl)
                    n532 = Divide(x=w913, y=3) -> (x/y=w915:dbl)
                    n533 = Format Value(format string="%#g", value (0)=w909) -> (output string=w910:string)  [unwired: 1 in]
                    n534 = To Word Integer(number=w915) -> (16bit integer=w914:i16)
                    n535 = Replace Array Subset(array=w916, new element=w910, index (row)=w914, index (col)=1) -> (w912:string[][])
                  }
                  frame True {
                  }
                }
                n536 = local write "Save Array"(w904) -> ()
              }
              frame #3 {
                n537 = local read "Save Array"() -> (w921:string[][])
                n538 = Array Size(array=w921) -> (size(s)=w926:i32[])
                n539 = Array Subset(array=w921, index (row)=0, index (col)=0, length (col)=3) -> (w922:string[][])  [unwired: 1 in]
                n540 = Index Array(array=w926, index=0) -> (element=w928:i32)
                n541 = Reshape Array(w922, w928) -> (w920:string[])
                n542 = Search 1D Array(1D array=w920, element="Width (um):") -> (index of element=w931:i32)  [unwired: 1 in]
                n543 = Equal?(x=w931, y=-1) -> (x = y?=w930:bool)
                n544 = case shown="False" w930 {
                  tunnel: w931 -> [w939 _]
                  tunnel: w921 -> [w938 w944]
                  tunnel: [w937 w944] -> w929
                  frame False {
                    n545 = local read "New: Width"() -> (w934:dbl)
                    n546 = Divide(x=w939, y=3) -> (x/y=w941:dbl)
                    n547 = To Word Integer(number=w941) -> (16bit integer=w940:i16)
                    n548 = Format Value(format string="%#g", value (0)=w934) -> (output string=w935:string)  [unwired: 1 in]
                    n549 = Replace Array Subset(array=w938, new element=w935, index (row)=w940, index (col)=1) -> (w937:string[][])
                  }
                  frame True {
                  }
                }
                n550 = local write "Save Array"(w929) -> ()
              }
              frame #4 {
                w954 = "Sample Temp (K):"
                n551 = local read "Save Array"() -> (w946:string[][])
                n552 = Array Size(array=w946) -> (size(s)=w951:i32[])
                n553 = Array Subset(array=w946, index (row)=0, index (col)=0, length (col)=3) -> (w947:string[][])  [unwired: 1 in]
                n554 = Index Array(array=w951, index=0) -> (element=w953:i32)
                n555 = Reshape Array(w947, w953) -> (w945:string[])
                n556 = Search 1D Array(1D array=w945, element=w954) -> (index of element=w957:i32)  [unwired: 1 in]
                n557 = Equal?(x=w957, y=-1) -> (x = y?=w956:bool)
                n558 = case shown="False" w956 {
                  tunnel: w946 -> [w966 w980]
                  tunnel: w957 -> [w963 _]
                  tunnel: [w962 w979] -> w955
                  tunnel: w945 -> [_ w982]
                  tunnel: w954 -> [_ w969]
                  frame False {
                    n559 = local read "New: Temp"() -> (w960:dbl)
                    n560 = Divide(x=w963, y=3) -> (x/y=w965:dbl)
                    n561 = Format Value(format string="%#g", value (0)=w960) -> (output string=w959:string)  [unwired: 1 in]
                    n562 = To Word Integer(number=w965) -> (16bit integer=w964:i16)
                    n563 = Replace Array Subset(array=w966, new element=w959, index (row)=w964, index (col)=1) -> (w962:string[][])
                  }
                  frame True {
                    n564 = local read "New: Temp"() -> (w971:dbl)
                    n565 = Search 1D Array(1D array=w982, element="Width (um):") -> (index of element=w976:i32)  [unwired: 1 in]
                    n566 = Divide(x=w976, y=3) -> (x/y=w977:dbl)
                    n567 = To Word Integer(number=w977) -> (16bit integer=w975:i16)
                    n568 = Format Value(format string="%#g", value (0)=w971) -> (output string=w970:string)  [unwired: 1 in]
                    n569 = Build Array(w969, w970) -> (w973:string[])
                    n570 = Increment(x=w975) -> (x+1=w974:i16)
                    n571 = Insert Into Array(array=w980, index (row)=w974, new element=w973) -> (w979:string[][])  [unwired: 1 in]
                  }
                }
                n572 = local write "Save Array"(w955) -> ()
              }
              frame #5 {
                w992 = "Mobility-Sat (cm^2/Vs):"
                n573 = local read "Save Array"() -> (w984:string[][])
                n574 = Array Size(array=w984) -> (size(s)=w989:i32[])
                n575 = Array Subset(array=w984, index (row)=0, index (col)=0, length (col)=3) -> (w985:string[][])  [unwired: 1 in]
                n576 = Index Array(array=w989, index=0) -> (element=w991:i32)
                n577 = Reshape Array(w985, w991) -> (w983:string[])
                n578 = Search 1D Array(1D array=w983, element=w992) -> (index of element=w995:i32)  [unwired: 1 in]
                n579 = Equal?(x=w995, y=-1) -> (x = y?=w994:bool)
                n580 = case shown="False" w994 {
                  tunnel: w984 -> [w1005 w1015]
                  tunnel: w995 -> [w1002 _]
                  tunnel: [w1001 w1014] -> w993
                  tunnel: w983 -> [_ w1012]
                  tunnel: w992 -> [_ w1010]
                  frame False {
                    n581 = local read "Re-Calculated Values Cluster"() -> (w998:T10)
                    n582 = Unbundle By Name(w998) -> ("Mobility-Sat"=w997:dbl)
                    n583 = Divide(x=w1002, y=3) -> (x/y=w1004:dbl)
                    n584 = To Word Integer(number=w1004) -> (16bit integer=w1003:i16)
                    n585 = Format Value(format string="%#g", value (0)=w997) -> (output string=w999:string)  [unwired: 1 in]
                    n586 = Replace Array Subset(array=w1005, new element=w999, index (row)=w1003, index (col)=1) -> (w1001:string[][])
                  }
                  frame True {
                    n587 = local read "Re-Calculated Values Cluster"() -> (w1009:T10)
                    n588 = Unbundle By Name(w1009) -> ("Mobility-Sat"=w1008:dbl)
                    n589 = Search 1D Array(1D array=w1012, element="Mobility (cm^2/Vs):") -> (index of element=w1018:i32)  [unwired: 1 in]
                    n590 = Divide(x=w1018, y=3) -> (x/y=w1019:dbl)
                    n591 = To Word Integer(number=w1019) -> (16bit integer=w1011:i16)
                    n592 = Format Value(format string="%#g", value (0)=w1008) -> (output string=w1013:string)  [unwired: 1 in]
                    n593 = Build Array(w1010, w1013) -> (w1017:string[])
                    n594 = Replace Array Subset(array=w1015, new element=w1017, index (row)=w1011) -> (w1014:string[][])  [unwired: 1 in]
                  }
                }
                n595 = local write "Save Array"(w993) -> ()
              }
              frame #6 {
                w1031 = "Mobility-Lin (cm^2/Vs):"
                n596 = local read "Save Array"() -> (w1022:string[][])
                n597 = Array Size(array=w1022) -> (size(s)=w1028:i32[])
                n598 = Array Subset(array=w1022, index (row)=0, index (col)=0, length (col)=3) -> (w1024:string[][])  [unwired: 1 in]
                n599 = Index Array(array=w1028, index=0) -> (element=w1030:i32)
                n600 = Reshape Array(w1024, w1030) -> (w1023:string[])
                n601 = Search 1D Array(1D array=w1023, element=w1031) -> (index of element=w1034:i32)  [unwired: 1 in]
                n602 = Equal?(x=w1034, y=-1) -> (x = y?=w1033:bool)
                n603 = case shown="True" w1033 {
                  tunnel: w1022 -> [w1044 w1052]
                  tunnel: w1034 -> [w1041 _]
                  tunnel: [w1040 w1051] -> w1032
                  tunnel: w1023 -> [_ w1050]
                  tunnel: w1031 -> [_ w1049]
                  frame False {
                    n604 = local read "Re-Calculated Values Cluster"() -> (w1037:T10)
                    n605 = Unbundle By Name(w1037) -> ("Moblitity-Lin"=w1036:dbl)
                    n606 = Divide(x=w1041, y=3) -> (x/y=w1043:dbl)
                    n607 = To Word Integer(number=w1043) -> (16bit integer=w1042:i16)
                    n608 = Format Value(format string="%#g", value (0)=w1036) -> (output string=w1038:string)  [unwired: 1 in]
                    n609 = Replace Array Subset(array=w1044, new element=w1038, index (row)=w1042, index (col)=1) -> (w1040:string[][])
                  }
                  frame True {
                    n610 = local read "Re-Calculated Values Cluster"() -> (w1048:T10)
                    n611 = Unbundle By Name(w1048) -> ("Moblitity-Lin"=w1047:dbl)
                    n612 = Search 1D Array(1D array=w1050, element="Mobility-Sat (cm^2/Vs):") -> (index of element=w1057:i32)  [unwired: 1 in]
                    n613 = Divide(x=w1057, y=3) -> (x/y=w1058:dbl)
                    n614 = To Word Integer(number=w1058) -> (16bit integer=w1056:i16)
                    n615 = Format Value(format string="%#g", value (0)=w1047) -> (output string=w1061:string)  [unwired: 1 in]
                    n616 = Build Array(w1049, w1061) -> (w1054:string[])
                    n617 = Increment(x=w1056) -> (x+1=w1055:i16)
                    n618 = Insert Into Array(array=w1052, index (row)=w1055, new element=w1054) -> (w1051:string[][])  [unwired: 1 in]
                  }
                }
                n619 = local write "Save Array"(w1032) -> ()
              }
              frame #7 {
                w1071 = "On/Off I-Sat:"
                n620 = local read "Save Array"() -> (w1062:string[][])
                n621 = Array Size(array=w1062) -> (size(s)=w1068:i32[])
                n622 = Array Subset(array=w1062, index (row)=0, index (col)=0, length (col)=3) -> (w1064:string[][])  [unwired: 1 in]
                n623 = Index Array(array=w1068, index=0) -> (element=w1070:i32)
                n624 = Reshape Array(w1064, w1070) -> (w1063:string[])
                n625 = Search 1D Array(1D array=w1063, element=w1071) -> (index of element=w1074:i32)  [unwired: 1 in]
                n626 = Equal?(x=w1074, y=-1) -> (x = y?=w1073:bool)
                n627 = case shown="True" w1073 {
                  tunnel: w1062 -> [w1084 w1093]
                  tunnel: w1074 -> [w1081 _]
                  tunnel: [w1080 w1094] -> w1072
                  tunnel: w1063 -> [_ w1091]
                  tunnel: w1071 -> [_ w1089]
                  frame False {
                    n628 = local read "Re-Calculated Values Cluster"() -> (w1077:T10)
                    n629 = Divide(x=w1081, y=3) -> (x/y=w1083:dbl)
                    n630 = Unbundle By Name(w1077) -> ("On/Off"=w1076:dbl)
                    n631 = To Word Integer(number=w1083) -> (16bit integer=w1082:i16)
                    n632 = Format Value(format string="%#g", value (0)=w1076) -> (output string=w1078:string)  [unwired: 1 in]
                    n633 = Replace Array Subset(array=w1084, new element=w1078, index (row)=w1082, index (col)=1) -> (w1080:string[][])
                  }
                  frame True {
                    n634 = local read "Re-Calculated Values Cluster"() -> (w1088:T10)
                    n635 = Unbundle By Name(w1088) -> ("On/Off"=w1087:dbl)
                    n636 = Search 1D Array(1D array=w1091, element="On/Off Current:") -> (index of element=w1097:i32)  [unwired: 1 in]
                    n637 = Divide(x=w1097, y=3) -> (x/y=w1098:dbl)
                    n638 = To Word Integer(number=w1098) -> (16bit integer=w1090:i16)
                    n639 = Format Value(format string="%#g", value (0)=w1087) -> (output string=w1092:string)  [unwired: 1 in]
                    n640 = Build Array(w1089, w1092) -> (w1096:string[])
                    n641 = Replace Array Subset(array=w1093, new element=w1096, index (row)=w1090) -> (w1094:string[][])  [unwired: 1 in]
                  }
                }
                n642 = local write "Save Array"(w1072) -> ()
              }
              frame #8 {
                w1110 = "Off I-Sat (A):"
                n643 = local read "Save Array"() -> (w1101:string[][])
                n644 = Array Size(array=w1101) -> (size(s)=w1107:i32[])
                n645 = Array Subset(array=w1101, index (row)=0, index (col)=0, length (col)=3) -> (w1103:string[][])  [unwired: 1 in]
                n646 = Index Array(array=w1107, index=0) -> (element=w1109:i32)
                n647 = Reshape Array(w1103, w1109) -> (w1102:string[])
                n648 = Search 1D Array(1D array=w1102, element=w1110) -> (index of element=w1113:i32)  [unwired: 1 in]
                n649 = Equal?(x=w1113, y=-1) -> (x = y?=w1112:bool)
                n650 = case shown="True" w1112 {
                  tunnel: w1101 -> [w1123 w1131]
                  tunnel: w1113 -> [w1120 _]
                  tunnel: [w1119 w1130] -> w1111
                  tunnel: w1102 -> [_ w1129]
                  tunnel: w1110 -> [_ w1128]
                  frame False {
                    n651 = local read "Re-Calculated Values Cluster"() -> (w1116:T10)
                    n652 = Unbundle By Name(w1116) -> ("Off Current"=w1115:dbl)
                    n653 = Divide(x=w1120, y=3) -> (x/y=w1122:dbl)
                    n654 = Format Value(format string="%#g", value (0)=w1115) -> (output string=w1117:string)  [unwired: 1 in]
                    n655 = To Word Integer(number=w1122) -> (16bit integer=w1121:i16)
                    n656 = Replace Array Subset(array=w1123, new element=w1117, index (row)=w1121, index (col)=1) -> (w1119:string[][])
                  }
                  frame True {
                    n657 = local read "Re-Calculated Values Cluster"() -> (w1127:T10)
                    n658 = Unbundle By Name(w1127) -> ("Off Current"=w1126:dbl)
                    n659 = Search 1D Array(1D array=w1129, element="On/Off I-Sat:") -> (index of element=w1136:i32)  [unwired: 1 in]
                    n660 = Divide(x=w1136, y=3) -> (x/y=w1137:dbl)
                    n661 = To Word Integer(number=w1137) -> (16bit integer=w1135:i16)
                    n662 = Format Value(format string="%#g", value (0)=w1126) -> (output string=w1140:string)  [unwired: 1 in]
                    n663 = Build Array(w1128, w1140) -> (w1133:string[])
                    n664 = Increment(x=w1135) -> (x+1=w1134:i16)
                    n665 = Insert Into Array(array=w1131, index (row)=w1134, new element=w1133) -> (w1130:string[][])  [unwired: 1 in]
                  }
                }
                n666 = local write "Save Array"(w1111) -> ()
              }
              frame #9 {
                w1142 = "Vt-Sat (V):"
                n667 = local read "Save Array"() -> (w1143:string[][])
                n668 = Array Size(array=w1143) -> (size(s)=w1148:i32[])
                n669 = Array Subset(array=w1143, index (row)=0, index (col)=0, length (col)=3) -> (w1144:string[][])  [unwired: 1 in]
                n670 = Index Array(array=w1148, index=0) -> (element=w1150:i32)
                n671 = Reshape Array(w1144, w1150) -> (w1141:string[])
                n672 = Search 1D Array(1D array=w1141, element=w1142) -> (index of element=w1153:i32)  [unwired: 1 in]
                n673 = Equal?(x=w1153, y=-1) -> (x = y?=w1152:bool)
                n674 = case shown="False" w1152 {
                  tunnel: w1143 -> [w1162 w1172]
                  tunnel: w1153 -> [w1158 _]
                  tunnel: [w1157 w1171] -> w1151
                  tunnel: w1142 -> [_ w1170]
                  tunnel: w1141 -> [_ w1169]
                  frame False {
                    n675 = local read "Re-Calculated Values Cluster"() -> (w1156:T10)
                    n676 = Unbundle By Name(w1156) -> ("Vt-Sat"=w1155:dbl)
                    n677 = Divide(x=w1158, y=3) -> (x/y=w1161:dbl)
                    n678 = To Word Integer(number=w1161) -> (16bit integer=w1160:i16)
                    n679 = Number To Fractional String(number=w1155) -> (F-format string=w1159:string)  [unwired: 3 in]
                    n680 = Replace Array Subset(array=w1162, new element=w1159, index (row)=w1160, index (col)=1) -> (w1157:string[][])
                  }
                  frame True {
                    n681 = local read "Re-Calculated Values Cluster"() -> (w1166:T10)
                    n682 = Unbundle By Name(w1166) -> ("Vt-Sat"=w1165:dbl)
                    n683 = Search 1D Array(1D array=w1169, element="Threshold V (V):") -> (index of element=w1168:i32)  [unwired: 1 in]
                    n684 = Divide(x=w1168, y=3) -> (x/y=w1175:dbl)
                    n685 = To Word Integer(number=w1175) -> (16bit integer=w1167:i16)
                    n686 = Format Value(format string="%#g", value (0)=w1165) -> (output string=w1178:string)  [unwired: 1 in]
                    n687 = Build Array(w1170, w1178) -> (w1174:string[])
                    n688 = Replace Array Subset(array=w1172, new element=w1174, index (row)=w1167) -> (w1171:string[][])  [unwired: 1 in]
                  }
                }
                n689 = local write "Save Array"(w1151) -> ()
              }
              frame #10 {
                n690 = disable-structure shown="Disabled" {
                  frame Disabled {
                    n691 = local read "Save Array"() -> (w1179:string[][])
                    n692 = Array Size(array=w1179) -> (size(s)=w1185:i32[])
                    n693 = Array Subset(array=w1179, index (row)=0, index (col)=0, length (col)=3) -> (w1181:string[][])  [unwired: 1 in]
                    n694 = Index Array(array=w1185, index=0) -> (element=w1187:i32)
                    n695 = Reshape Array(w1181, w1187) -> (w1180:string[])
                    n696 = Search 1D Array(1D array=w1180, element="VT-Lin (V):") -> (index of element=w1190:i32)  [unwired: 1 in]
                    n697 = Equal?(x=w1190, y=-1) -> (x = y?=w1189:bool)
                    n698 = case shown="False" w1189 {
                      tunnel: w1179 -> [w1199 w1202]
                      tunnel: w1190 -> [w1196 _]
                      tunnel: [w1195 w1202] -> w1188
                      frame False {
                        n699 = Divide(x=w1196, y=3) -> (x/y=w1198:dbl)
                        n700 = To Word Integer(number=w1198) -> (16bit integer=w1197:i16)
                        n701 = Format Value(format string="%#g") -> (output string=w1193:string)  [unwired: 2 in]
                        n702 = Replace Array Subset(array=w1199, new element=w1193, index (row)=w1197, index (col)=1) -> (w1195:string[][])
                      }
                      frame True {
                      }
                    }
                    n703 = local write "Save Array"(w1188) -> ()
                  }
                  frame Enabled {
                  }
                }
              }
              frame #11 {
                w1203 = "STS-Sat (V/decade):"
                n704 = local read "Save Array"() -> (w1205:string[][])
                n705 = Array Size(array=w1205) -> (size(s)=w1210:i32[])
                n706 = Array Subset(array=w1205, index (row)=0, index (col)=0, length (col)=3) -> (w1206:string[][])  [unwired: 1 in]
                n707 = Index Array(array=w1210, index=0) -> (element=w1212:i32)
                n708 = Reshape Array(w1206, w1212) -> (w1204:string[])
                n709 = Search 1D Array(1D array=w1204, element=w1203) -> (index of element=w1215:i32)  [unwired: 1 in]
                n710 = Equal?(x=w1215, y=-1) -> (x = y?=w1214:bool)
                n711 = case shown="True" w1214 {
                  tunnel: w1205 -> [w1225 w1233]
                  tunnel: w1215 -> [w1222 _]
                  tunnel: [w1221 w1234] -> w1213
                  tunnel: w1204 -> [_ w1232]
                  tunnel: w1203 -> [_ w1231]
                  frame False {
                    n712 = local read "Re-Calculated Values Cluster"() -> (w1217:T10)
                    n713 = Unbundle By Name(w1217) -> ("STS"=w1218:dbl)
                    n714 = Divide(x=w1222, y=3) -> (x/y=w1224:dbl)
                    n715 = To Word Integer(number=w1224) -> (16bit integer=w1223:i16)
                    n716 = Format Value(format string="%#g", value (0)=w1218) -> (output string=w1219:string)  [unwired: 1 in]
                    n717 = Replace Array Subset(array=w1225, new element=w1219, index (row)=w1223, index (col)=1) -> (w1221:string[][])
                  }
                  frame True {
                    n718 = local read "Re-Calculated Values Cluster"() -> (w1228:T10)
                    n719 = Unbundle By Name(w1228) -> ("STS"=w1229:dbl)
                    n720 = Search 1D Array(1D array=w1232, element="S.T.S. (V/decade):") -> (index of element=w1237:i32)  [unwired: 1 in]
                    n721 = Divide(x=w1237, y=3) -> (x/y=w1238:dbl)
                    n722 = To Word Integer(number=w1238) -> (16bit integer=w1230:i16)
                    n723 = Format Value(format string="%#g", value (0)=w1229) -> (output string=w1241:string)  [unwired: 1 in]
                    n724 = Build Array(w1231, w1241) -> (w1236:string[])
                    n725 = Replace Array Subset(array=w1233, new element=w1236, index (row)=w1230) -> (w1234:string[][])  [unwired: 1 in]
                  }
                }
                n726 = local write "Save Array"(w1213) -> ()
              }
              frame #12 {
                w1242 = "Trap Density-VT (Traps/Vcm^2):"
                n727 = local read "Save Array"() -> (w1244:string[][])
                n728 = Array Size(array=w1244) -> (size(s)=w1249:i32[])
                n729 = Array Subset(array=w1244, index (row)=0, index (col)=0, length (col)=3) -> (w1245:string[][])  [unwired: 1 in]
                n730 = Index Array(array=w1249, index=0) -> (element=w1251:i32)
                n731 = Reshape Array(w1245, w1251) -> (w1243:string[])
                n732 = Search 1D Array(1D array=w1243, element=w1242) -> (index of element=w1254:i32)  [unwired: 1 in]
                n733 = Equal?(x=w1254, y=-1) -> (x = y?=w1253:bool)
                n734 = case shown="True" w1253 {
                  tunnel: w1244 -> [w1264 w1271]
                  tunnel: w1254 -> [w1260 _]
                  tunnel: [w1259 w1272] -> w1252
                  tunnel: w1243 -> [_ w1270]
                  tunnel: w1242 -> [_ w1269]
                  frame False {
                    n735 = local read "Re-Calculated Values Cluster"() -> (w1257:T10)
                    n736 = Unbundle By Name(w1257) -> ("Trap Density-VT"=w1256:dbl)
                    n737 = Divide(x=w1260, y=3) -> (x/y=w1263:dbl)
                    n738 = To Word Integer(number=w1263) -> (16bit integer=w1262:i16)
                    n739 = Format Value(format string="%#g", value (0)=w1256) -> (output string=w1261:string)  [unwired: 1 in]
                    n740 = Replace Array Subset(array=w1264, new element=w1261, index (row)=w1262, index (col)=1) -> (w1259:string[][])
                  }
                  frame True {
                    n741 = local read "Re-Calculated Values Cluster"() -> (w1268:T10)
                    n742 = Unbundle By Name(w1268) -> ("Trap Density-VT"=w1267:dbl)
                    n743 = Search 1D Array(1D array=w1270, element="STS-Sat (V/decade):") -> (index of element=w1277:i32)  [unwired: 1 in]
                    n744 = Divide(x=w1277, y=3) -> (x/y=w1276:dbl)
                    n745 = To Word Integer(number=w1276) -> (16bit integer=w1278:i16)
                    n746 = Format Value(format string="%#g", value (0)=w1267) -> (output string=w1273:string)  [unwired: 1 in]
                    n747 = Build Array(w1269, w1273) -> (w1280:string[])
                    n748 = Increment(x=w1278) -> (x+1=w1279:i16)
                    n749 = Insert Into Array(array=w1271, index (row)=w1279, new element=w1280) -> (w1272:string[][])  [unwired: 1 in]
                  }
                }
                n750 = local write "Save Array"(w1252) -> ()
              }
              frame #13 {
                w1282 = "Trap Density-STS (Traps/Vcm^2):"
                n751 = local read "Save Array"() -> (w1284:string[][])
                n752 = Array Size(array=w1284) -> (size(s)=w1289:i32[])
                n753 = Array Subset(array=w1284, index (row)=0, index (col)=0, length (col)=3) -> (w1285:string[][])  [unwired: 1 in]
                n754 = Index Array(array=w1289, index=0) -> (element=w1291:i32)
                n755 = Reshape Array(w1285, w1291) -> (w1283:string[])
                n756 = Search 1D Array(1D array=w1283, element=w1282) -> (index of element=w1294:i32)  [unwired: 1 in]
                n757 = Equal?(x=w1294, y=-1) -> (x = y?=w1293:bool)
                n758 = case shown="True" w1293 {
                  tunnel: w1284 -> [w1304 w1311]
                  tunnel: w1294 -> [w1301 _]
                  tunnel: [w1300 w1312] -> w1292
                  tunnel: w1283 -> [_ w1310]
                  tunnel: w1282 -> [_ w1309]
                  frame False {
                    n759 = local read "Re-Calculated Values Cluster"() -> (w1297:T10)
                    n760 = Unbundle By Name(w1297) -> ("Trap Density-STS"=w1296:dbl)
                    n761 = Divide(x=w1301, y=3) -> (x/y=w1303:dbl)
                    n762 = To Word Integer(number=w1303) -> (16bit integer=w1302:i16)
                    n763 = Format Value(format string="%#g", value (0)=w1296) -> (output string=w1298:string)  [unwired: 1 in]
                    n764 = Replace Array Subset(array=w1304, new element=w1298, index (row)=w1302, index (col)=1) -> (w1300:string[][])
                  }
                  frame True {
                    n765 = local read "Re-Calculated Values Cluster"() -> (w1308:T10)
                    n766 = Unbundle By Name(w1308) -> ("Trap Density-STS"=w1307:dbl)
                    n767 = Search 1D Array(1D array=w1310, element="Trap Density-VT (Traps/Vcm^2):") -> (index of element=w1317:i32)  [unwired: 1 in]
                    n768 = Divide(x=w1317, y=3) -> (x/y=w1318:dbl)
                    n769 = To Word Integer(number=w1318) -> (16bit integer=w1316:i16)
                    n770 = Format Value(format string="%#g", value (0)=w1307) -> (output string=w1321:string)  [unwired: 1 in]
                    n771 = Build Array(w1309, w1321) -> (w1314:string[])
                    n772 = Increment(x=w1316) -> (x+1=w1315:i16)
                    n773 = Insert Into Array(array=w1311, index (row)=w1315, new element=w1314) -> (w1312:string[][])  [unwired: 1 in]
                  }
                }
                n774 = local write "Save Array"(w1292) -> ()
              }
            }
            n775 = local read "New: Temp"() -> (w829:dbl)
            n776 = local read "New: Width"() -> (w830:dbl)
            n777 = local read "New: Length"() -> (w832:dbl)
            n778 = local read "Index"() -> (w831:string)
            n779 = To Single Precision Float(number=w829) -> (single precision float=w846:sgl)
            n780 = Number To Decimal String(number=w846) -> (decimal integer string=w841:string)  [unwired: 1 in]
            n781 = To Single Precision Float(number=w830) -> (single precision float=w845:sgl)
            n782 = To Single Precision Float(number=w832) -> (single precision float=w844:sgl)
            n783 = Strip Path(path=w828) -> (stripped path=w833:path)  [unwired: 1 out]
            n784 = Number To Decimal String(number=w844) -> (decimal integer string=w839:string)  [unwired: 1 in]
            n785 = Number To Decimal String(number=w845) -> (decimal integer string=w838:string)  [unwired: 1 in]
            n786 = Concatenate Strings("_", w841, "K") -> (w843:string)
            n787 = call "Build Text"("Temp"=w843, "Index"=w831, "Length"=w839, "Width"=w838) -> ("Result"=w837:string)  [unwired: 10 in, 1 out]
            n788 = Path To String(path=w833) -> (string=w835:string)
            n789 = Concatenate Strings(w835, "\\", w837) -> (w836:string)
            n790 = String To Path(string=w836) -> (path=w827:path)
          }
          frame #1 {
            n791 = flat-sequence {
              tunnel: w1325 -> [w1327]
              tunnel: w1324 -> [w1326]
              tunnel: [w1326] -> w1323
              tunnel: w1323 -> [w1333]
              tunnel: w1322 -> [w1332]
              frame #0 {
                n792 = Equal?(x=w1327, y=w1326) -> (x = y?=w1328:bool)
                n793 = case shown="False" w1328 {
                  tunnel: w1327 -> [w1331 _]
                  tunnel: w1326 -> [w1330 _]
                  frame False {
                    n794 = Move(source path=w1331, 9:TRUE, 10:w1330) -> ()  [unwired: 2 in, 3 out]
                  }
                  frame True {
                  }
                }
              }
              frame #1 {
                n795 = local write "Transfer File"(w1333) -> ()
                n796 = call-poly <vilib>:"Write To Spreadsheet File.vi"("2D data"=w1332, "file path (dialog if empty)"=w1333) -> ()  [unwired: 6 in, 1 out]
              }
            }
          }
        }
        n797 = Cluster To Array(cluster=w817) -> (array=w816:bool[])
        n798 = Boolean Array To Number(Boolean array=w816) -> (number=w815:u32)
        n799 = Equal To 0?(x=w815) -> (x = 0?=w814:bool)
        n800 = case shown="True" w814 {
          tunnel: [MegaAwesome_States."Read Data" w821] -> w813
          tunnel: w812 -> [_ w825]
          frame False {
          }
          frame True {
            n801 = Unbundle By Name(w825) -> ("Save Next"=w824:bool)
            n802 = Select(t=MegaAwesome_States."No Event", s=w824, f=MegaAwesome_States."Next File") -> (s? t:f=w821:T3)
          }
        }
      }
      frame "Exit" {
      }
      frame "Save Lines" {
        n803 = Build Path(base path=w1337, name or relative path="ROI") -> (appended path=w1340:path)
        n804 = call <vilib>:"Check if File or Folder Exists.vi"("path"=w1340) -> ("file or folder exists?"=w1338:bool, "dup path"=w1341:path)  [unwired: 8 in, 1 out]
        n805 = case shown="False" w1338 {
          tunnel: w1341 -> [w1349 w1350]
          tunnel: [w1348 w1350] -> w1345
          frame False {
            n806 = Create Folder(path (use dialog)=w1349) -> (created path=w1348:path)  [unwired: 2 in, 2 out]
          }
          frame True {
          }
        }
        n807 = local read "Index"() -> (w1336:string)
        n808 = property on="Image Out" class="ImageControl"() -> ("ROI"=w1342:T13)  [unwired: 2 in, 2 out]
        n809 = Build Path(base path=w1345, name or relative path=w1336) -> (appended path=w1344:path)
        n810 = Flatten To String(anything=w1342) -> (data string=w1343:string)  [unwired: 3 in, 2 out]
        n811 = Write to Text File(file (use dialog)=w1344, text=w1343) -> ()  [unwired: 2 in, 3 out]
      }
      frame "Export" {
        n812 = flat-sequence {
          frame #0 {
            n813 = stacked-sequence {
              frame #0 {
                n814 = local read "Independant Variable:"() -> (w1353:string)
                n815 = Equal?(x=w1353, y="Length (um):") -> (x = y?=w1354:bool)
                n816 = case shown="True" w1354 {
                  frame False {
                  }
                  frame True {
                    n817 = local write "X Axis Display Type"("1") -> ()
                    n818 = local write "Opj X Axis"("2") -> ()
                  }
                }
              }
              frame #1 {
                n819 = local read "Independant Variable:"() -> (w1358:string)
                n820 = Equal?(x=w1358, y="Sample Temp (K):") -> (x = y?=w1359:bool)
                n821 = case shown="True" w1359 {
                  frame False {
                  }
                  frame True {
                    n822 = local write "X Axis Display Type"("1") -> ()
                    n823 = local write "Opj X Axis"("1") -> ()
                  }
                }
              }
              frame #2 {
                n824 = local read "Independant Variable:"() -> (w1363:string)
                n825 = Equal?(x=w1363, y="Mobility-Sat (cm^2/Vs):") -> (x = y?=w1364:bool)
                n826 = case shown="True" w1364 {
                  frame False {
                  }
                  frame True {
                    n827 = local write "X Axis Display Type"("2") -> ()
                    n828 = local write "Opj X Axis"("2") -> ()
                  }
                }
              }
              frame #3 {
                n829 = local read "Independant Variable:"() -> (w1368:string)
                n830 = Equal?(x=w1368, y="Mobility-Lin (cm^2/Vs):") -> (x = y?=w1369:bool)
                n831 = case shown="True" w1369 {
                  frame False {
                  }
                  frame True {
                    n832 = local write "X Axis Display Type"("2") -> ()
                    n833 = local write "Opj X Axis"("2") -> ()
                  }
                }
              }
              frame #4 {
                n834 = local read "Independant Variable:"() -> (w1373:string)
                n835 = Equal?(x=w1373, y="On/Off I-Sat:") -> (x = y?=w1374:bool)
                n836 = case shown="True" w1374 {
                  frame False {
                  }
                  frame True {
                    n837 = local write "X Axis Display Type"("2") -> ()
                    n838 = local write "Opj X Axis"("2") -> ()
                  }
                }
              }
              frame #5 {
                n839 = local read "Independant Variable:"() -> (w1378:string)
                n840 = Equal?(x=w1378, y="Off I-Sat (A):") -> (x = y?=w1379:bool)
                n841 = case shown="True" w1379 {
                  frame False {
                  }
                  frame True {
                    n842 = local write "X Axis Display Type"("2") -> ()
                    n843 = local write "Opj X Axis"("2") -> ()
                  }
                }
              }
              frame #6 {
                n844 = local read "Independant Variable:"() -> (w1383:string)
                n845 = Equal?(x=w1383, y="Vt-Sat (V):") -> (x = y?=w1384:bool)
                n846 = case shown="True" w1384 {
                  frame False {
                  }
                  frame True {
                    n847 = local write "X Axis Display Type"("1") -> ()
                    n848 = local write "Opj X Axis"("1") -> ()
                  }
                }
              }
              frame #7 {
                n849 = local read "Independant Variable:"() -> (w1388:string)
                n850 = Equal?(x=w1388, y="STS-Sat (V/decade):") -> (x = y?=w1389:bool)
                n851 = case shown="True" w1389 {
                  frame False {
                  }
                  frame True {
                    n852 = local write "X Axis Display Type"("1") -> ()
                    n853 = local write "Opj X Axis"("1") -> ()
                  }
                }
              }
              frame #8 {
                n854 = local read "Independant Variable:"() -> (w1393:string)
                n855 = Equal?(x=w1393, y="Trap Density-VT (Traps/Vcm^2):") -> (x = y?=w1394:bool)
                n856 = case shown="True" w1394 {
                  frame False {
                  }
                  frame True {
                    n857 = local write "X Axis Display Type"("2") -> ()
                    n858 = local write "Opj X Axis"("2") -> ()
                  }
                }
              }
              frame #9 {
                n859 = local read "Independant Variable:"() -> (w1398:string)
                n860 = Equal?(x=w1398, y="Trap Density-STS (Traps/Vcm^2):") -> (x = y?=w1399:bool)
                n861 = case shown="True" w1399 {
                  frame False {
                  }
                  frame True {
                    n862 = local write "X Axis Display Type"("2") -> ()
                    n863 = local write "Opj X Axis"("2") -> ()
                  }
                }
              }
            }
          }
          frame #1 {
            n864 = local read "Transfer Folder"() -> (w1407:path)
            n865 = Build Path(base path=w1407, name or relative path="Stats") -> (appended path=w1408:path)
            n866 = local read "Origin Project File"() -> (w1419:path)
            n867 = call <vilib>:"Check if File or Folder Exists.vi"("path"=w1408) -> ("file or folder exists?"=w1423:bool, "dup path"=w1422:path)  [unwired: 8 in, 1 out]
            n868 = call <userlib>:"OA_ConnectToOrigin.vi"() -> ("error out"=w1420:errorcluster, "Origin.IOApplication"=w1421:refnum<k7>)  [unwired: 8 in]
            n869 = case shown="False" w1423 {
              tunnel: w1422 -> [w1596 w1597]
              tunnel: [w1595 w1597] -> w1406
              frame False {
                n870 = Create Folder(path (use dialog)=w1596) -> (created path=w1595:path)  [unwired: 2 in, 2 out]
              }
              frame True {
              }
            }
            n871 = call "File Dialog"("start path"=w1408) -> ("selected path"=w1410:path)  [unwired: 11 in, 3 out]
            n872 = call <userlib>:"OA_Load.vi"("error in (no error)"=w1420, "Path"=w1419, "Origin.IOApplication"=w1421) -> ("error out"=w1417:errorcluster, "Origin.IOApplication"=w1418:refnum<k7>)  [unwired: 1 out]
            n873 = call "OAExecute.vi"("script"="document -m 3;", "Error IO"=w1417, "Origin.IOApplication"=w1418) -> ("Error IO Out"=w1415:errorcluster, "Origin.IOApplication"=w1416:refnum<k7>)  [unwired: 1 in, 1 out]
            n874 = local read "Independant Variable:"() -> (w1403:string)
            n875 = stacked-sequence {
              tunnel: w1407 -> [w1434 w1464 w1476 w1498 w1518 w1539 w1560 w1583]
              tunnel: w1406 -> [w1435 w1463 w1477 w1497 w1519 w1540 w1561 w1584]
              tunnel: w1416 -> [w1437 w1461 w1479 w1500 w1521 w1542 w1563 w1586]
              tunnel: w1415 -> [w1436 w1462 w1478 w1499 w1520 w1541 w1562 w1585]
              tunnel: [_ _ _ _ _ _ _ w1581] -> w1405
              tunnel: [_ _ _ _ _ _ _ w1582] -> w1404
              tunnel: w1403 -> [w1433 w1454 w1475 w1496 w1517 w1538 w1559 w1580]
              frame #0 {
                n876 = local read "X Axis Display Type"() -> (w1425:string)
                n877 = local read "Opj X Axis"() -> (w1430:string)
                n878 = Concatenate Strings("window -a MOBLGraph;\nlayer.x.type=", w1430, "; layer.x.label.numFormat = ", w1425, "; Y3 = 1; X3 = 1;", "window -a MOBLTable;\nwindow -s TV;") -> (w1428:string)
                n879 = call "Param_Analysis_7_24b_JW.vi"("Independant Variable"=w1433, "error in (no error)"=w1436, "Data Folder"=w1434, "Parameter String"="Mobility-Lin (cm^2/Vs):", "Parameter Name"="Mobility-Lin", "Stats Folder"=w1435) -> ("error out"=w1439:errorcluster, "Output Array"=w1441:string[][], "Variables"=w1432:T27)  [unwired: 2 in, 1 out]
                n880 = call "Origin_Export_7_27a_JW.vi"("Input Conditions"=w1432, "Analysis Array"=w1441, "error in (no error)"=w1439, "Parameter Worksheet Name"="[MOBLTable]Mobilities", "Parameter Folder Script"="pe_cd \"Mobility-Lin\";", "Origin.IOApplication"=w1437) -> ("error out"=w1438:errorcluster, "reference out"=w1440:refnum<k7>)  [unwired: 3 in, 1 out]
                n881 = call "OAExecute.vi"("script"=w1428, "Error IO"=w1438, "Origin.IOApplication"=w1440) -> ()  [unwired: 1 in, 3 out]
              }
              frame #1 {
                n882 = local read "X Axis Display Type"() -> (w1446:string)
                n883 = local read "Opj X Axis"() -> (w1451:string)
                n884 = Concatenate Strings("window -a MOBSGraph;\nlayer.x.type=", w1451, "; layer.x.label.numFormat = ", w1446, "; Y3 = 1; X3 = 1;", "window -a MOBSTable;\nwindow -s TV;") -> (w1449:string)
                n885 = call "Param_Analysis_7_24b_JW.vi"("Independant Variable"=w1454, "error in (no error)"=w1462, "Data Folder"=w1464, "Parameter String"="Mobility-Sat (cm^2/Vs):", "Parameter Name"="Mobility-Sat", "Stats Folder"=w1463) -> ("error out"=w1457:errorcluster, "Output Array"=w1455:string[][], "Variables"=w1453:T27)  [unwired: 2 in, 1 out]
                n886 = call "Origin_Export_7_27a_JW.vi"("Input Conditions"=w1453, "Analysis Array"=w1455, "error in (no error)"=w1457, "Parameter Worksheet Name"="[MOBSTable]Mobilities", "Parameter Folder Script"="pe_cd \"Mobility-Sat\";", "Origin.IOApplication"=w1461) -> ("error out"=w1456:errorcluster, "reference out"=w1458:refnum<k7>)  [unwired: 3 in, 1 out]
                n887 = call "OAExecute.vi"("script"=w1449, "Error IO"=w1456, "Origin.IOApplication"=w1458) -> ()  [unwired: 1 in, 3 out]
              }
              frame #2 {
                n888 = local read "X Axis Display Type"() -> (w1467:string)
                n889 = local read "Opj X Axis"() -> (w1472:string)
                n890 = Concatenate Strings("window -a NSTSGraph;\nlayer.x.type=", w1472, "; layer.x.label.numFormat = ", w1467, "; Y3 = 1; X3 = 1;", "window -a NSTSTable;\nwindow -s TV;") -> (w1470:string)
                n891 = call "Param_Analysis_7_24b_JW.vi"("Independant Variable"=w1475, "error in (no error)"=w1478, "Data Folder"=w1476, "Parameter String"="Trap Density-STS (Traps/Vcm^2):", "Parameter Name"="Trap Density-STS", "Stats Folder"=w1477) -> ("error out"=w1482:errorcluster, "Output Array"=w1480:string[][], "Variables"=w1474:T27)  [unwired: 2 in, 1 out]
                n892 = call "Origin_Export_7_27a_JW.vi"("Input Conditions"=w1474, "Analysis Array"=w1480, "error in (no error)"=w1482, "Parameter Worksheet Name"="[NSTSTable]Trap Densities", "Parameter Folder Script"="pe_cd \"N-STS\";", "Origin.IOApplication"=w1479) -> ("error out"=w1481:errorcluster, "reference out"=w1483:refnum<k7>)  [unwired: 3 in, 1 out]
                n893 = call "OAExecute.vi"("script"=w1470, "Error IO"=w1481, "Origin.IOApplication"=w1483) -> ()  [unwired: 1 in, 3 out]
              }
              frame #3 {
                n894 = local read "X Axis Display Type"() -> (w1488:string)
                n895 = local read "Opj X Axis"() -> (w1493:string)
                n896 = call "Param_Analysis_7_24b_JW.vi"("Independant Variable"=w1496, "error in (no error)"=w1499, "Data Folder"=w1498, "Parameter String"="Trap Density-VT (Traps/Vcm^2):", "Parameter Name"="Trap Density-Vt", "Stats Folder"=w1497) -> ("error out"=w1503:errorcluster, "Output Array"=w1501:string[][], "Variables"=w1495:T27)  [unwired: 2 in, 1 out]
                n897 = Concatenate Strings("window -a NVtGraph;\nlayer.x.type=", w1493, "; layer.x.label.numFormat = ", w1488, "; Y3 = 1; X3 = 1;", "window -a NVtTable;\nwindow -s TV;") -> (w1491:string)
                n898 = call "Origin_Export_7_27a_JW.vi"("Input Conditions"=w1495, "Analysis Array"=w1501, "error in (no error)"=w1503, "Parameter Worksheet Name"="[NVTTable]Trap Densities", "Parameter Folder Script"="pe_cd \"N-Vt\";", "Origin.IOApplication"=w1500) -> ("error out"=w1502:errorcluster, "reference out"=w1504:refnum<k7>)  [unwired: 3 in, 1 out]
                n899 = call "OAExecute.vi"("script"=w1491, "Error IO"=w1502, "Origin.IOApplication"=w1504) -> ()  [unwired: 1 in, 3 out]
              }
              frame #4 {
                n900 = local read "X Axis Display Type"() -> (w1509:string)
                n901 = local read "Opj X Axis"() -> (w1514:string)
                n902 = Concatenate Strings("window -a OffIGraph;\nlayer.x.type=", w1514, "; layer.x.label.numFormat = ", w1509, "; Y3 = 1; X3 = 1;", "window -a OffITable;\nwindow -s TV;") -> (w1512:string)
                n903 = call "Param_Analysis_7_24b_JW.vi"("Independant Variable"=w1517, "error in (no error)"=w1520, "Data Folder"=w1518, "Parameter String"="Off I-Sat (A):", "Parameter Name"="Off I-Sat", "Stats Folder"=w1519) -> ("error out"=w1524:errorcluster, "Output Array"=w1522:string[][], "Variables"=w1516:T27)  [unwired: 2 in, 1 out]
                n904 = call "Origin_Export_7_27a_JW.vi"("Input Conditions"=w1516, "Analysis Array"=w1522, "error in (no error)"=w1524, "Parameter Worksheet Name"="[OffItable]OffCurrents", "Parameter Folder Script"="pe_cd \"OffI-Sat\";", "Origin.IOApplication"=w1521) -> ("error out"=w1523:errorcluster, "reference out"=w1525:refnum<k7>)  [unwired: 3 in, 1 out]
                n905 = call "OAExecute.vi"("script"=w1512, "Error IO"=w1523, "Origin.IOApplication"=w1525) -> ()  [unwired: 1 in, 3 out]
              }
              frame #5 {
                n906 = local read "X Axis Display Type"() -> (w1530:string)
                n907 = local read "Opj X Axis"() -> (w1535:string)
                n908 = Concatenate Strings("window -a OnOffGraph;\nlayer.x.type=", w1535, "; layer.x.label.numFormat = ", w1530, "; Y3 = 1; X3 = 1;", "window -a OnOffTable;\nwindow -s TV;") -> (w1533:string)
                n909 = call "Param_Analysis_7_24b_JW.vi"("Independant Variable"=w1538, "error in (no error)"=w1541, "Data Folder"=w1539, "Parameter String"="On/Off I-Sat:", "Parameter Name"="OnOff Ratio", "Stats Folder"=w1540) -> ("error out"=w1545:errorcluster, "Output Array"=w1543:string[][], "Variables"=w1537:T27)  [unwired: 2 in, 1 out]
                n910 = call "Origin_Export_7_27a_JW.vi"("Input Conditions"=w1537, "Analysis Array"=w1543, "error in (no error)"=w1545, "Parameter Worksheet Name"="[OnOffTable]On/Off Ratios", "Parameter Folder Script"="pe_cd \"OnOff-Ratio\";", "Origin.IOApplication"=w1542) -> ("error out"=w1544:errorcluster, "reference out"=w1546:refnum<k7>)  [unwired: 3 in, 1 out]
                n911 = call "OAExecute.vi"("script"=w1533, "Error IO"=w1544, "Origin.IOApplication"=w1546) -> ()  [unwired: 1 in, 3 out]
              }
              frame #6 {
                n912 = local read "X Axis Display Type"() -> (w1551:string)
                n913 = local read "Opj X Axis"() -> (w1556:string)
                n914 = call "Param_Analysis_7_24b_JW.vi"("Independant Variable"=w1559, "error in (no error)"=w1562, "Data Folder"=w1560, "Parameter String"="STS-Sat (V/decade):", "Parameter Name"="STS-Sat", "Stats Folder"=w1561) -> ("error out"=w1566:errorcluster, "Output Array"=w1564:string[][], "Variables"=w1558:T27)  [unwired: 2 in, 1 out]
                n915 = Concatenate Strings("window -a SGraph;\nlayer.x.type=", w1556, "; layer.x.label.numFormat = ", w1551, "; Y3 = 1; X3 = 1;", "window -a STable;\nwindow -s TV;") -> (w1554:string)
                n916 = call "Origin_Export_7_27a_JW.vi"("Input Conditions"=w1558, "Analysis Array"=w1564, "error in (no error)"=w1566, "Parameter Worksheet Name"="[STable]Threshold Swing", "Parameter Folder Script"="pe_cd \"STS-Sat\";", "Origin.IOApplication"=w1563) -> ("error out"=w1565:errorcluster, "reference out"=w1567:refnum<k7>)  [unwired: 3 in, 1 out]
                n917 = call "OAExecute.vi"("script"=w1554, "Error IO"=w1565, "Origin.IOApplication"=w1567) -> ()  [unwired: 1 in, 3 out]
              }
              frame #7 {
                n918 = local read "X Axis Display Type"() -> (w1572:string)
                n919 = local read "Opj X Axis"() -> (w1577:string)
                n920 = Concatenate Strings("window -a VtGraph;\nlayer.x.type=", w1577, "; layer.x.label.numFormat = ", w1572, "; Y3 = 1; X3 = 1;", "window -a VtTable;\nwindow -s TV;") -> (w1575:string)
                n921 = call "Param_Analysis_7_24b_JW.vi"("Independant Variable"=w1580, "error in (no error)"=w1585, "Data Folder"=w1583, "Parameter String"="Vt-Sat (V):", "Parameter Name"="Vt-Sat", "Stats Folder"=w1584) -> ("error out"=w1589:errorcluster, "Output Array"=w1587:string[][], "Variables"=w1579:T27)  [unwired: 2 in, 1 out]
                n922 = call "Origin_Export_7_27a_JW.vi"("Input Conditions"=w1579, "Analysis Array"=w1587, "error in (no error)"=w1589, "Parameter Worksheet Name"="[VtTable]Threshold Voltages", "Parameter Folder Script"="pe_cd \"Vt-Sat\";", "Origin.IOApplication"=w1586) -> ("error out"=w1588:errorcluster, "reference out"=w1590:refnum<k7>)  [unwired: 3 in, 1 out]
                n923 = call "OAExecute.vi"("script"=w1575, "Error IO"=w1588, "Origin.IOApplication"=w1590) -> ("Error IO Out"=w1581:errorcluster, "Origin.IOApplication"=w1582:refnum<k7>)  [unwired: 1 in, 1 out]
              }
            }
            n924 = Path To String(path=w1410) -> (string=w1409:string)
            n925 = call "OAExecute.vi"("script"="pe_cd /; ", "Error IO"=w1405, "Origin.IOApplication"=w1404) -> ("Error IO Out"=w1411:errorcluster, "Origin.IOApplication"=w1412:refnum<k7>)  [unwired: 1 in, 1 out]
            n926 = call <userlib>:"OASaveProject.vi"("path"=w1409, "Error IO"=w1411, "Origin.IOApplication"=w1412) -> ()  [unwired: 3 out]
          }
        }
      }
    }
    "Current State" <- w19
    "Folder Index" <- w12
    n927 = Wait (ms)(milliseconds to wait=w6) -> ()  [unwired: 1 out]
    n928 = Equal?(x=w21, y=MegaAwesome_States."Exit") -> (x = y?=w22:bool)
  }
